vi "slow_control_2_15.vi"() -> ()   [LabVIEW 2018]
uses:
  4623b864-5764-45c6-9cb2-3e18237880ca.vi
  fa57f61f-0bb9-49ac-92eb-fcb40add4dbb.vi
  <vilib>/DAQmx/read.llb/DAQmx Read (Analog 1D DBL NChan 1Samp).vi
  ffb0d1b3-ef19-4e2e-b36e-7277177ef4b3.vi
  9a1acc8a-69db-4048-9e4c-bb07d66d2422.vi
  <vilib>/DAQmx/create/channels.llb/DAQmx Create Channel (AI-Voltage-Basic).vi
  <vilib>/DAQmx/create/channels.llb/DAQmx Create Channel (AI-Current-Basic).vi
  <vilib>/DAQmx/create/channels.llb/DAQmx Create Channel (AI-Temperature-RTD).vi
  <vilib>/DAQmx/miscellaneous.llb/DAQmx Fill In Error Info.vi
  <vilib>/Utility/file.llb/Read Delimited Spreadsheet (string).vi
  <instrlib>/Lake Shore 335/Lake Shore 335.lvlib
  <instrlib>/CAEN PSM/CAEN PSM.lvlib
  <resource>/objmgr/daqmx.rc
panel:
  out "Heater":dbl
  out "Coldhead":dbl
  out "Cycle number":i32
  out "Alarm state":bool
  out "Timestamp last \nmeasured (UPS)":timestamp
  out "Auto-clear":bool
  in  "Auto-clear data?":bool
  in  "Clear data":bool
  in  "Clear data every N cycles":dbl
  in  "N samples":i32=30
  out "Average Flow (SLPM)":dbl caption="Flow (SLPM)"
  out "CAEN Ch. Names":string[](array[string])
  in  "Cycles to execute":dbl=5.0 format="%#_13g"
  out "Detector Pressure":dbl
  in  "N samples":i32=20
  in  "Allows tabs on \nfront panel":T1(tab)
  in  "Anode ch.":enum16{"1", "2", "3", "4"}(ring)=enum."3"
  in  "CAEN unit selector":enum16{"CAEN 1", "CAEN 2"}(ring)
  in  "Multipliers":dbl[](array[numeric])=[1.0, 1.0, 1.0, 1.0, 1.0, 1.0, 1.0, 1.0]
  in  "Offsets\nsubtracted":dbl[](array[numeric])=[0.0, 0.0, 0.0, 0.0, 0.0, 0.0, 0.0, 0.0]
  in  "Channel Names (9207, ai8:15)":string[](array[string])=["i0", "i1", "i2", "i3", "i4", "i5", "i6", "i7"] caption="\"Other\""
  in  "Flow meter input:":u16(ring)=3 items=["v0", "v1", "v2", "v3", "v4", "v5", "v6", "v7"]
  in  "Detector pressure input:":u16(ring) items=["v0", "v1", "v2", "v3", "v4", "v5", "v6", "v7"]
  in  "Channel Names (9207, ai0:7)":string[](array[string])=["v0", "v1", "v2", "v3", "v4", "v5", "v6", "v7"] caption="\"Other\""
  in  "Multipliers":dbl[](array[numeric])=[1.0, 1.0, 1.0, 1.0, 1.0, 1.0, 1.0, 1.0]
  in  "Offsets\nsubtracted":dbl[](array[numeric])=[0.0, 0.0, 0.0, 0.0, 0.0, 0.0, 0.0, 0.0]
  in  "Voltage channels":tag[](array[tag])=["9207/ai0", "9207/ai1", "9207/ai2", "9207/ai3", "9207/ai4", "9207/ai5", "9207/ai6", "9207/ai7"]
  in  "COM-port CAEN 1":refnum<visa-resource-name>
  in  "COM-port CAEN 2":refnum<visa-resource-name>
  in  "Run lakeshore?":bool
  in  "ID Query":bool
  in  "COM-port LakeShore":refnum<visa-resource-name>
  in  "PID settings":cluster{"P":dbl, "I":dbl, "D":dbl}={"P"=50.0, "I"=20.0, "D"=120.0}
  in  "Setpoint (°C)":dbl=-100.0 format="%.1f"
  in  "Heater range":u16(ring) items=["Off", "Low (On)", "Medium", "High"]
  in  "Current channels":tag[](array[tag])=["9207/ai8", "9207/ai9", "9207/ai10", "9207/ai11", "9207/ai12", "9207/ai13", "9207/ai14", "9207/ai15"]
  in  "Channel Names (CAEN)":string[](array[string])=["PMT 1", "PMT 2", "Anode", "Cathode", "Top gate", "Bottom gate", "Other 1", "Other 2"]
  in  "RTD Type":i32(ring)=10071 items=["Pt3750"=12481, "Pt3851"=10071, "Pt3911"=12482, "Pt3916"=10069, "Pt3920"=10053, "Pt3928"=12483, "Custom"=10137]
  in  "Module 1 channels (slot 1)":tag[](array[tag])=["cDAQ2Mod2/ai0", "cDAQ2Mod2/ai1", "cDAQ2Mod2/ai2", "cDAQ2Mod2/ai3", "cDAQ2Mod2/ai4", "cDAQ2Mod2/ai5", "cDAQ2Mod2/ai6", "cDAQ2Mod2/ai7"]
  in  "Current Excitation Source":i32(ring)=10200 items=["Internal"=10200, "External"=10167, "None"=10230]
  in  "Resistance Configuration":i32(ring)=3 items=["2-Wire"=2, "3-Wire"=3, "4-Wire"=4]
  in  "R (T = 0°C):":dbl=100.0
  in  "B":dbl
  in  "A":dbl
  in  "C":dbl
  in  "Module 2 channels (slot 2)":tag[](array[tag])=["cDAQ2Mod3/ai0", "cDAQ2Mod3/ai1", "cDAQ2Mod3/ai2", "cDAQ2Mod3/ai3", "cDAQ2Mod3/ai4", "cDAQ2Mod3/ai5", "cDAQ2Mod3/ai6", "cDAQ2Mod3/ai7"]
  in  "Shut off heater \nif Alarm is active":bool=TRUE
  in  "Re-save headers":bool
  in  "Resistance Configuration":i32(ring)=2 items=["2-Wire"=2, "3-Wire"=3, "4-Wire"=4]
  in  "Module 3 channels":tag[](array[tag])
  in  "RTD Type":i32(ring)=12481 items=["Pt3750"=12481, "Pt3851"=10071, "Pt3911"=12482, "Pt3916"=10069, "Pt3920"=10053, "Pt3928"=12483, "Custom"=10137]
  in  "R (T = 0°C)":dbl=100.0 format="%0.2f"
  out "PT1000 data":dbl[](array[numeric]) format="%0.2f"
  out "9207 (V; A) Converted":dbl[](array[numeric])
  out "9216 #1 (°C)":dbl[](array[numeric])
  out "9216 #2 (°C)":dbl[](array[numeric])
  out "Raw readouts (V, mA)":dbl[](array[numeric]) format="%0.2f"
  out "Det.P input #":i32
  out "Flow input #":i32
  out "PT100 data":dbl[](array[numeric]) format="%0.2f"
  in  "\"Sound\" alarm":bool
  in  "Sound alarm\nFrequency (Hz)":dbl=1680.0
  in  "Send status email now":bool
  out "Email error":i32
  out "source":string
  in  "Number of Bonus lines":i32=1
  out "Names (optional)":string[](array[string])
  in  "Send daily email?":bool=TRUE
  in  "Phone numbers":string[](array[string])
  out "Alarm (or test) message":string
  in  "Alarm\nMaster switch":bool
  in  "Repeat Alarm SMS\nevery N minutes":dbl=15.0
  in  "Test alarm":bool
  out "Warning":bool
  in  "UPS":bool
  in  "UPS Voltage \nLower Threshold":dbl=220.0
  out "NI mod 2&3 status":bool
  in  "NI mod 2&3":bool
  in  "NI mod 1":bool
  in  "CAEN 2":bool
  in  "CAEN 1":bool
  in  "LakeShore":bool
  out "Det. P. warning":bool
  out "Boolean 6":bool
  out "Boolean 5":bool
  out "Boolean 4":bool
  out "Boolean 3":bool
  out "Boolean 2":bool
  out "Boolean":bool
  in  "T 6":bool
  in  "T 5":bool
  in  "T 4":bool
  in  "T 3":bool
  in  "T 2":bool
  in  "T 1":bool
  in  "Detector Pressure":bool
  in  "Overpressure threshold":dbl
  in  "Underpressure threshold":dbl
  out "Comm. status":bool
  in  "High Temp threshold":dbl format="%#_13g"
  in  "Low Temp threshold":dbl format="%#_13g"
  out "LakeShore status":bool
  out "NI mod1 (P) status":bool
  out "CAEN 1 status":bool
  out "CAEN 2 status":bool
  out "Initialization status":bool
  out "Minimum input voltage measured":dbl
  out "Alarm active 2":bool
  out "SMS error":string
  out "Status email preview":string
  in  "Send status email at time:":string="14:00"
  in  "Email Addresses":string[](array[string])
  in  "return address":string="xamsups@gmail.com"
  in  "Ignore Initialization Errors":bool=TRUE caption="Ignore init. errors?"
  out "NI 9226":errorcluster
  in  "HV Channel status":string="Click the button to request the latest High Voltage channel status.\nView another channel with the arrows, or typing 0 through 3."
  out "CAEN 1":T2(array[cluster])
  out "CAEN 2":T2(array[cluster])
  in  "Query HV status":bool
  in  "\"code\"":string="Google this"
  in  "String 7":string="A checkmark means \"No error\" and false. A red X means an error occurred"
  out "\"status\"":bool
  in  "\"source\"":string="This may show two things: the latest executed VI in the task chain, in reverse order, or: which VI produced an error, with a short description. If the error can't easily be resolved, google the code."
  out "NI 9216 x2":errorcluster
  out "CAEN 1":errorcluster
  out "CAEN 2":errorcluster
  out "Lakeshore":errorcluster
  out "NI 9207":errorcluster
  in  "Temperature channel selector":u16(ring) items=["0"=0, "1"=1, "2"=2, "3"=3, "4"=4, "5"=5, "6"=6, "7"=7, "Average"=666]
  out "Heater power (%)":cluster{timestamp[], dbl[]}[](graph)
  out "Flow (SLPM)":cluster{timestamp[], dbl[]}[](graph)
  out "9207 (ai 0:7, Volts)":cluster{timestamp[], dbl[]}[](graph)
  out "Phase Diagram":cluster{"X":dbl, "Y":dbl}[](graph)
  out "Temperature (9216 0:15, °C)":cluster{timestamp[], dbl[]}[](graph)
  in  "Pause?":bool
  out "Integrated Flow (SL)":dbl
  in  "Reset?":bool
  out "LakeShore readings":dbl[](array[numeric])
  out "Detector Temperature (9226, 0:7, °C)":cluster{"X":dbl, "Y":dbl}[](graph)
  out "Temp A":dbl
  out "Temp B":dbl
  in  "Temperature Channel Selector":u16(ring) items=["0", "1", "2", "3", "4", "5", "6", "7"]
  out "Historical Large Phase Diagram":cluster{dbl[], dbl[]}[](graph)
  out "Large Phase Diagram":cluster{"X":dbl, "Y":dbl}[](graph)
  in  "Temperature Channel Selector":u16(ring) items=["0"=0, "1"=1, "2"=2, "3"=3, "4"=4, "5"=5, "6"=6, "7"=7, "Average"=666]
  in  "Scale.Range:Minimum 8":dbl
  in  "Scale.Range:Maximum 8":dbl=4000.0
  in  "Scale.Range:Minimum 7":dbl
  in  "Scale.Range:Maximum 7":dbl=4000.0
  in  "Scale.Range:Minimum 6":dbl=-3000.0
  in  "Scale.Range:Maximum 6":dbl
  in  "Scale.Range:Minimum 5":dbl
  in  "Scale.Range:Maximum 5":dbl=3000.0
  in  "Scale.Range:Minimum 4":dbl=-5000.0
  in  "Scale.Range:Maximum 4":dbl
  in  "Scale.Range:Maximum 3":dbl=4000.0
  in  "Scale.Range:Minimum 3":dbl
  in  "Scale.Range:Maximum 2":dbl=1000.0
  in  "Scale.Range:Minimum 2":dbl
  out "CAEN 1.1":dbl(knob) scale=0.0..1000.0
  out "CAEN 1.1":string
  in  "Scale.Range:Maximum":dbl=1000.0
  in  "Scale.Range:Minimum":dbl
  out "CAEN 2.3 2":string
  out "CAEN 2.2 2":string
  out "Channel Names":string[](array[string])
  out "CAEN 2.3":dbl(knob) scale=0.0..4000.0
  out "CAEN 2.2":dbl(knob) scale=0.0..4000.0
  out "CAEN 2.1":string
  out "CAEN 2.0":string
  out "CAEN 1.3":string
  out "CAEN 1.2":string
  out "CAEN 1.0":string
  out "Channel Names":string[](array[string])
  in  "Set to zero":bool
  out "CAEN 2.1":dbl(knob)
  out "CAEN 2.0":dbl(knob) scale=0.0..3000.0
  in  "Apply Voltage":bool
  in  "VSet (V)":dbl[](array[numeric])
  in  "IMax (uA)":dbl[](array[numeric])
  in  "VMax (V)":dbl[](array[numeric])
  out "CAEN 1.3":dbl(knob)
  out "CAEN 1.2":dbl(knob) scale=0.0..4000.0
  out "CAEN 1.0":dbl(knob) scale=0.0..1000.0
  out "Vmon (V)":dbl[](array[numeric])
  out "IMon (uA)":dbl[](array[numeric])
  in  "Read CAEN units \nevery N cycles":i16=120
  in  "Reset anode\nperiodically?":bool
  in  "Kill every Y minutes":i32=10
  in  "Keep off for X seconds":i32=10
  out "?":bool
  out "Killed":bool
  out "Restarted":bool
  out "Anode timers":timestamp[](array[timestamp])
  out "Seconds until \nanode autokill":dbl format="%.2g"
  out "Seconds until \nanode reset":dbl format="%.2g"
  out "9207 (ai 8:15, Amperes)":cluster{timestamp[], dbl[]}[](graph)
  in  "Kill voltage":bool
  in  "stop":bool
  out "Voltages":dbl[](array[numeric])
  out "Started up?":bool
  out "TOBA appended":dbl[][](array[numeric])
  in  "Read T every N cycles":i32=2
  out "Time until next cycle":dbl format="%.3g"
  in  "Time per cycle (s)":i32=2 caption="Time Target (s)"
  # "<- Proof of concept for New/Old T + New P"
  # "Remove ^this^ array, just for testing and takes up lots of resources"
  # "Moving averages"
  # "NI 9216 Temperature settings"
  # "CAEN settings"
  # "NI 9207 Voltage settings"
  # "If RTD type is custom,\nspecify the Callendar-\nVan Dusen parameters"
  # "Anode connected to:"
  # "Channel:"
  # "NI 9207 Current settings"
  # "Lakeshore settings"
  # "NI 9226 Temperature settings"
  # "Gain (P) (XX.X)"
  # "Reset (I) (XX.X)"
  # "Rate (D) (X.X%)"
  # "Alarm indicators and arms"
  # "Detector Thresholds"
  # "Daily status email"
  # "SMS and sound alarm"
  # "Alarm conditions"
  # "Temperature channels:"
  # "Uninterruptable Power Supply"
  # "Task information"
  # "High Voltage channel status"
  # "How-to"
  # "Data"
  # "Scale:"
  # "to"
  # "to"
  # "Scale:"
  # "Time of last reset"
  # "Time of last reactivation"
  # "to"
  # "Scale:"
  # "to"
  # "Scale:"
  # "Settings"
  # "Scale:"
  # "to"
  # "Scale:"
  # "to"
  # "Scale:"
  # "to"
  # "to"
  # "Scale:"
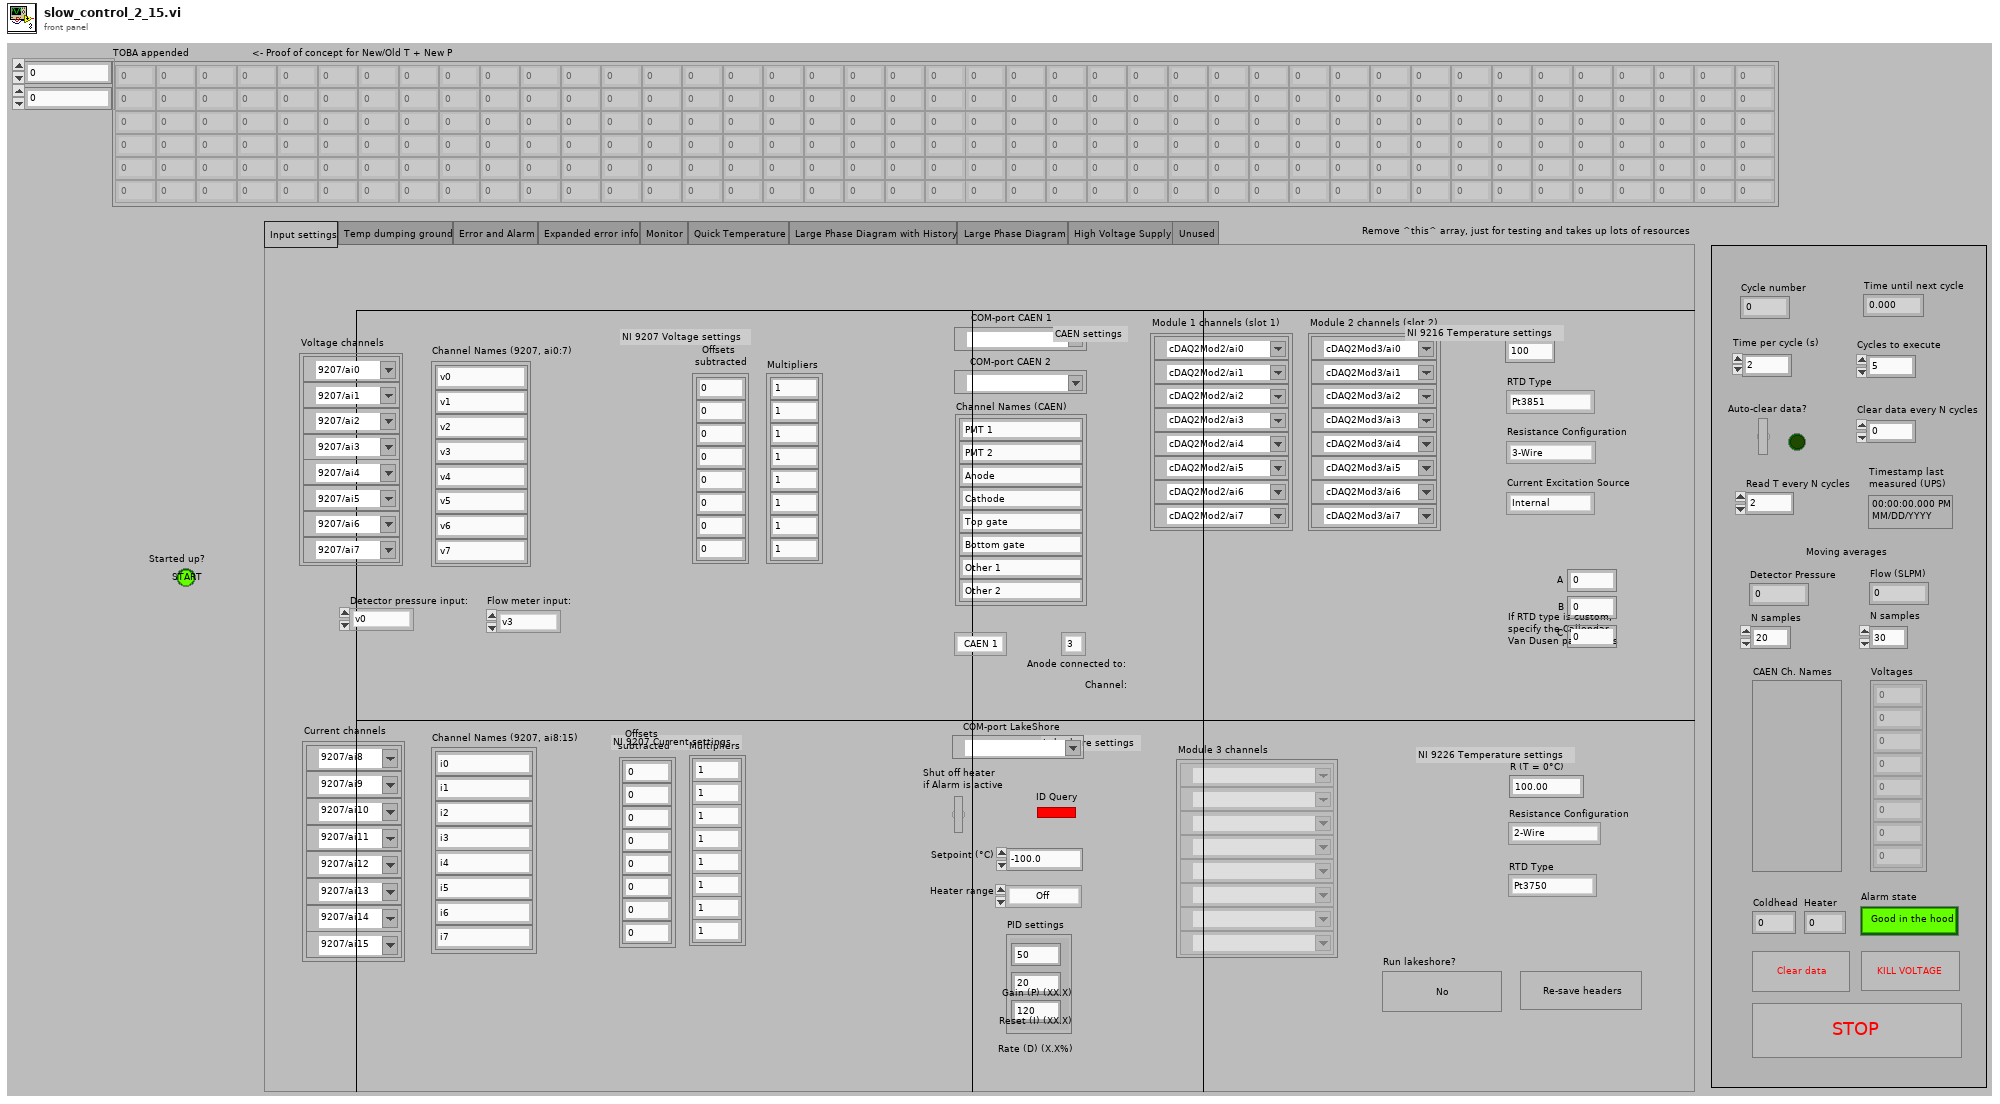
[diagram p1: front panel]
types:
  T1 = enum32{"Input settings", "Temp dumping ground", "Error and Alarm", "Expanded error info", "Monitor", "Quick Temperature", "Large Phase Diagram with History", "Large Phase Diagram", "High Voltage Supply", "Unused"}
  T2 = cluster{"ON":bool, "RUP":bool, "RDW":bool, "OVC":bool, "OVV":bool, "UNV":bool, "MAXV":bool, "TRIP":bool, "OVP":bool, "OVT":bool, "DIS":bool, "KILL":bool, "ILK":bool, "NOCAL":bool}[]
  T3 = cluster{"Baud Rate":u32, "Parity":u16, "Data Bits":u16, "Stop Bits":u16, "Flow Control":u16}
  T4 = cluster{"task out":refnum<k21>, "error out":errorcluster}
  T5 = cluster{"VISA resource name out":refnum<visa-resource-name>, "error out":errorcluster}
  T6 = cluster{"VISA resource name out":refnum<visa-resource-name>, "Board address":u8, "NChannels":u8}
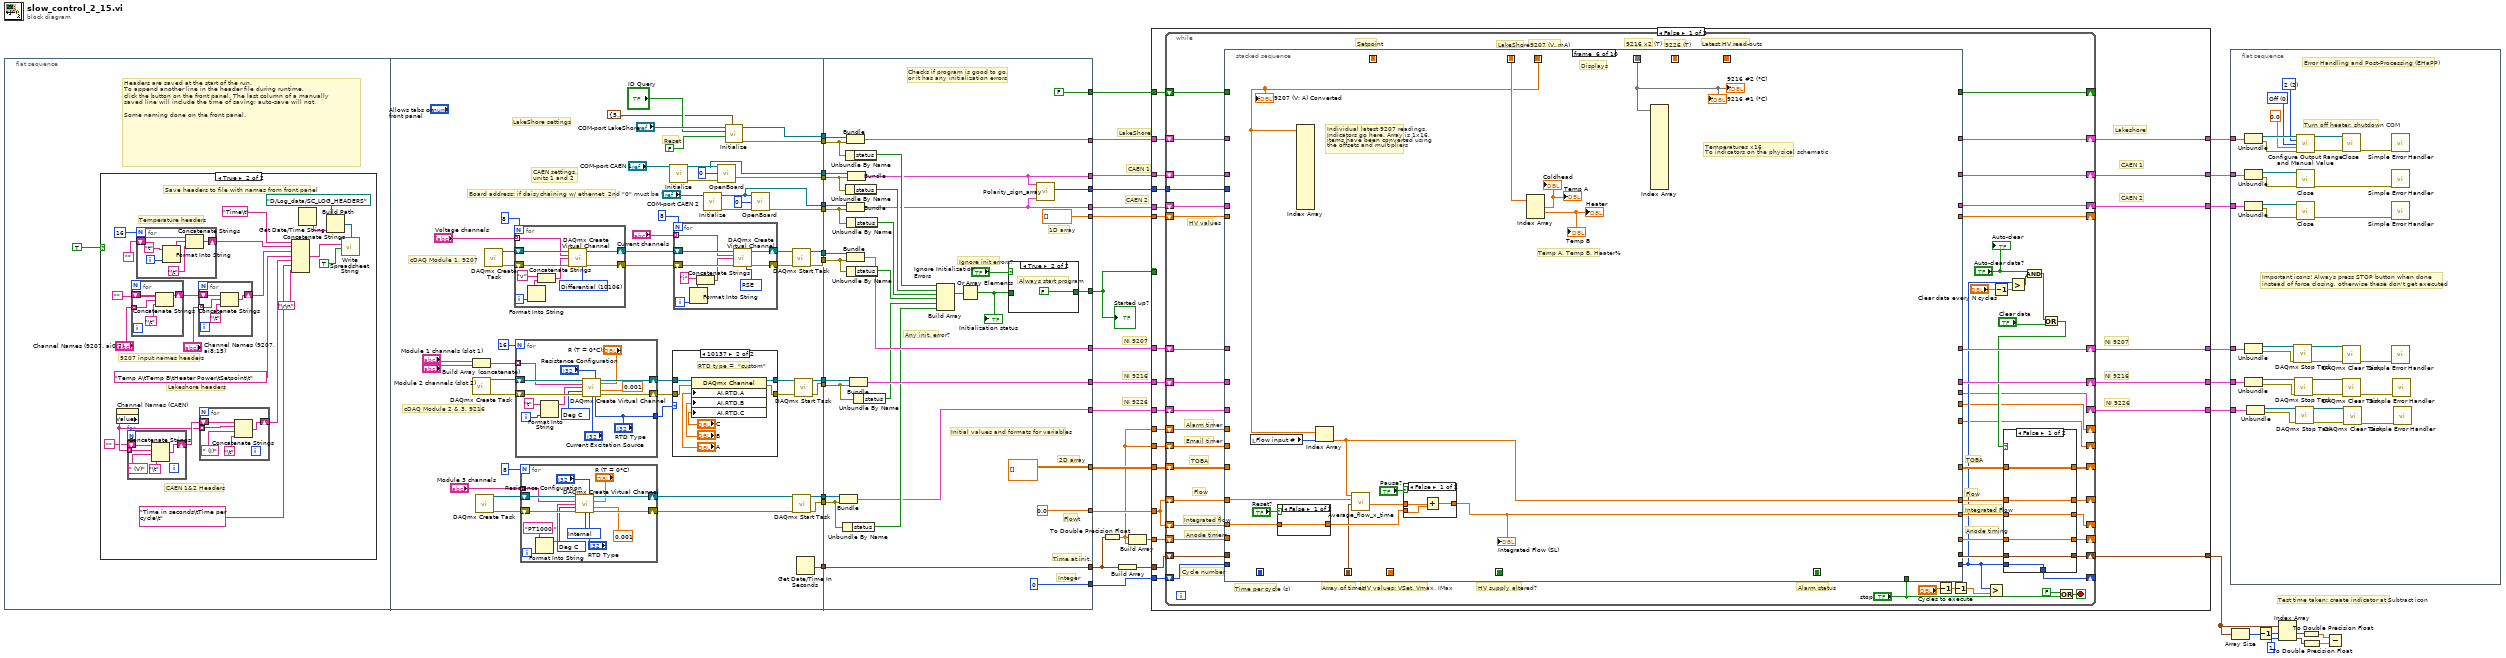
[diagram p0: block diagram]
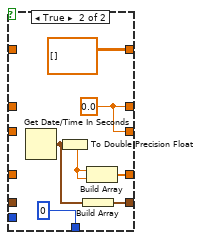
[diagram p2: hidden frame]
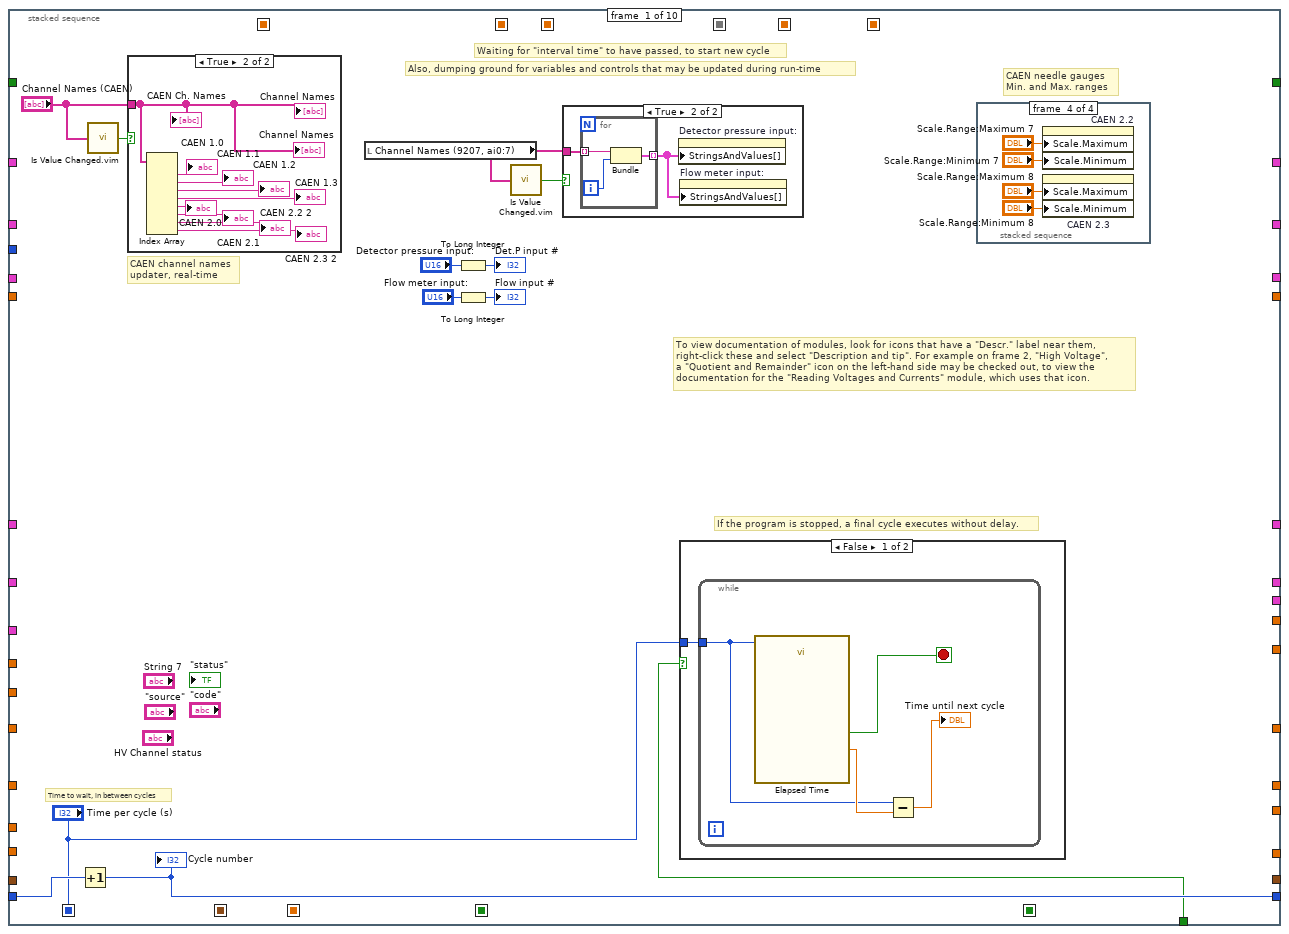
[diagram p3: hidden frame]
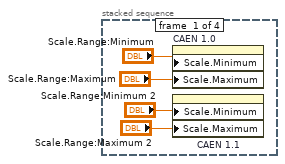
[diagram p6: hidden frame]
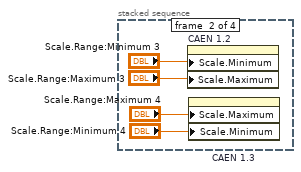
[diagram p7: hidden frame]
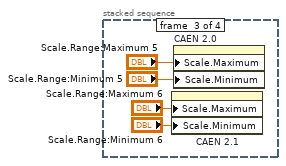
[diagram p8: hidden frame]
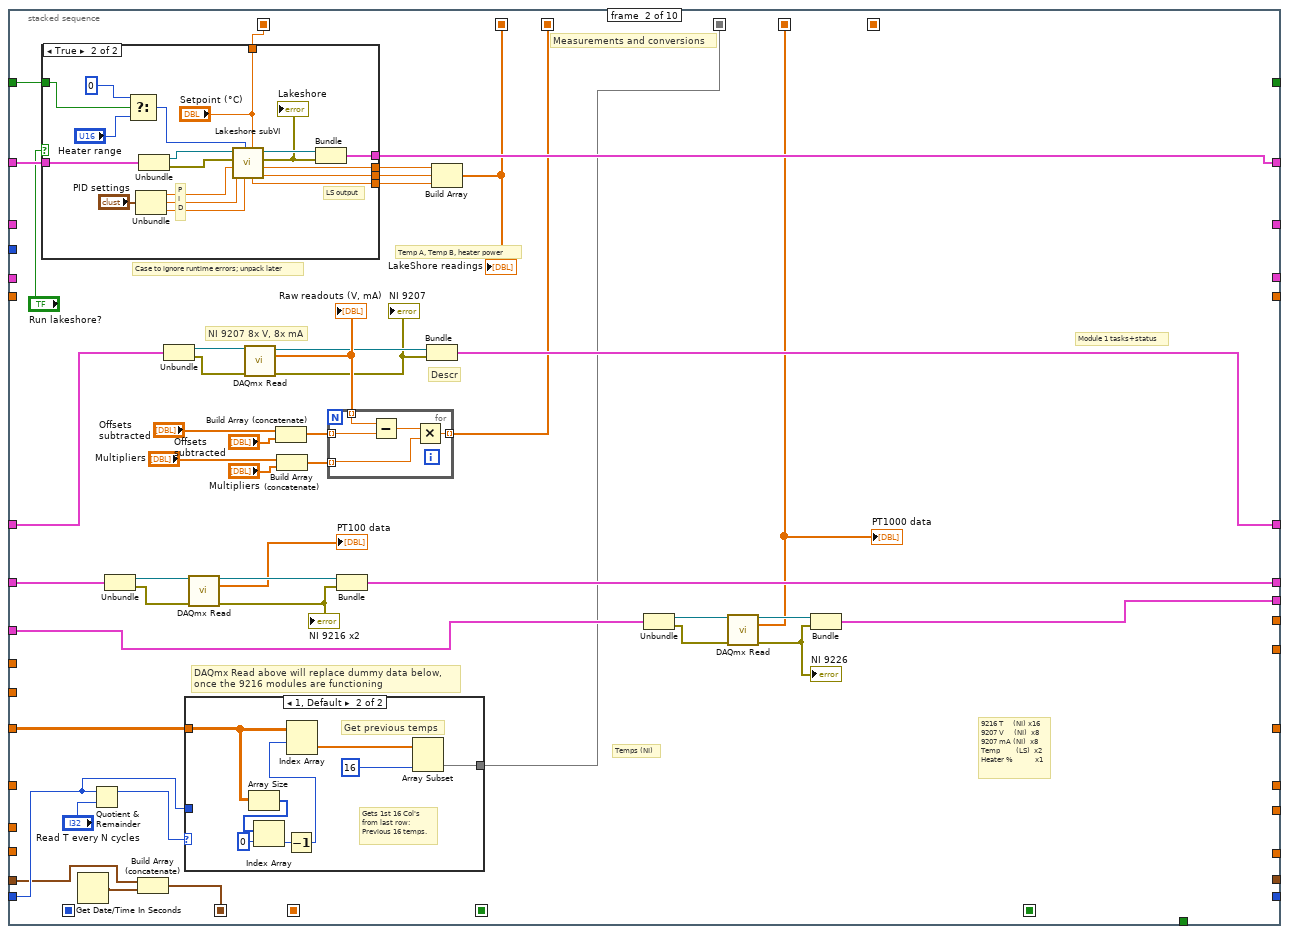
[diagram p10: hidden frame]
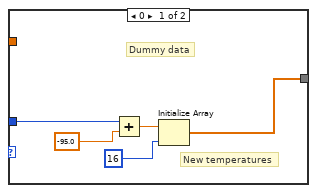
[diagram p11: hidden frame]
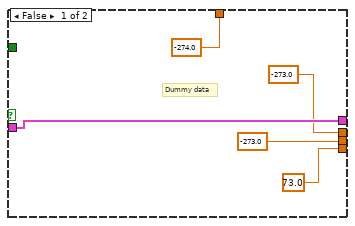
[diagram p12: hidden frame]
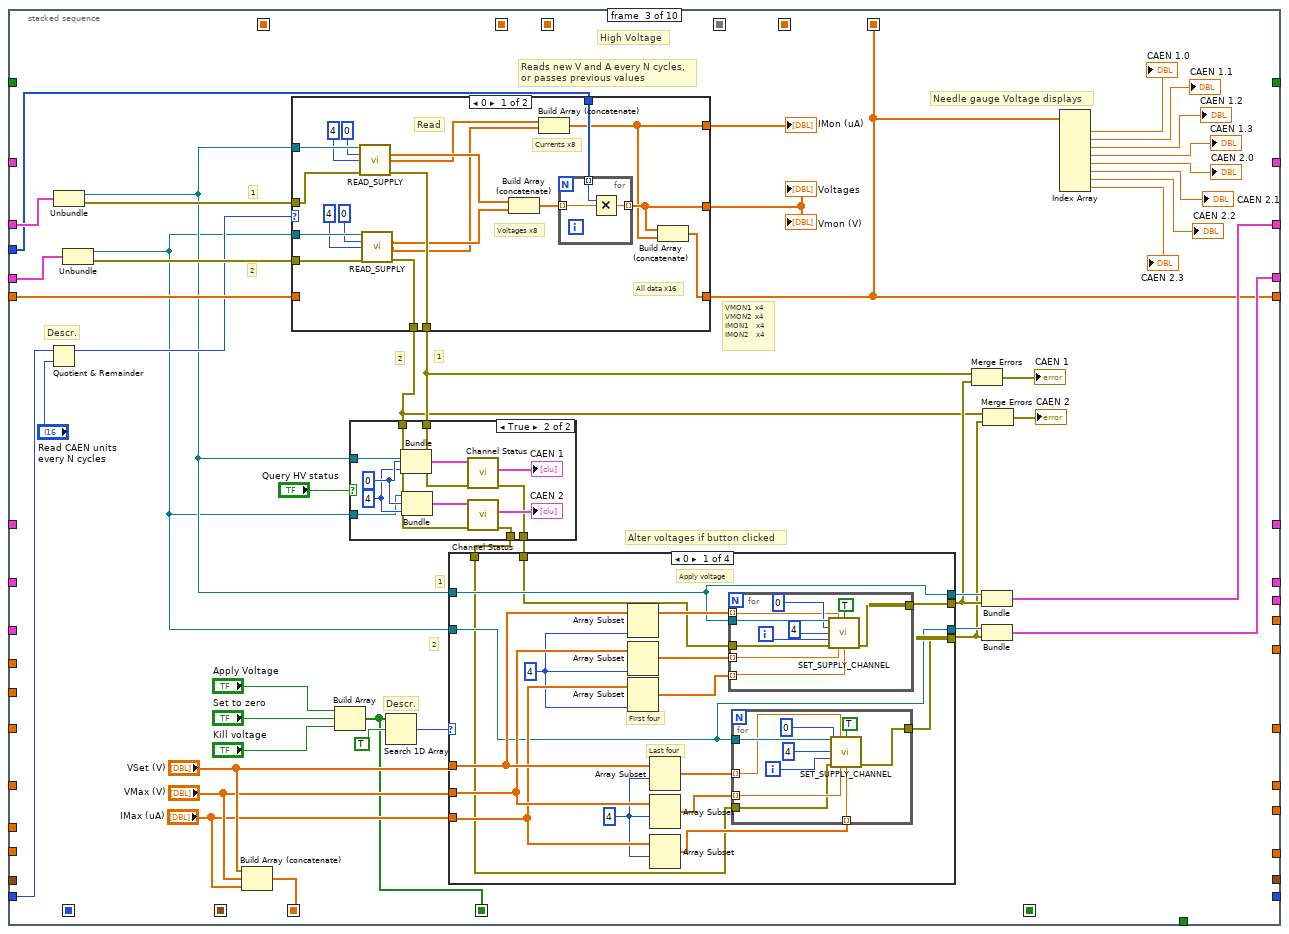
[diagram p13: hidden frame]
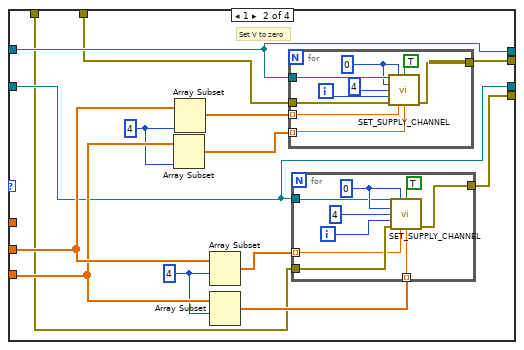
[diagram p15: hidden frame]
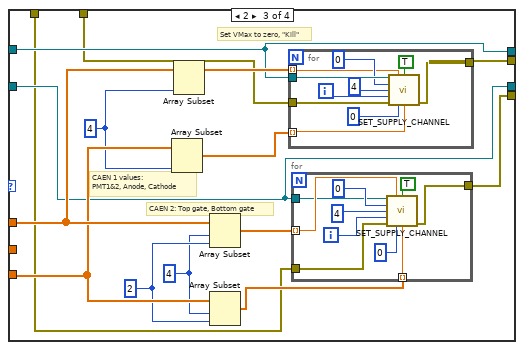
[diagram p16: hidden frame]
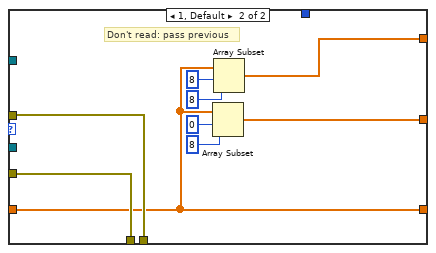
[diagram p18: hidden frame]
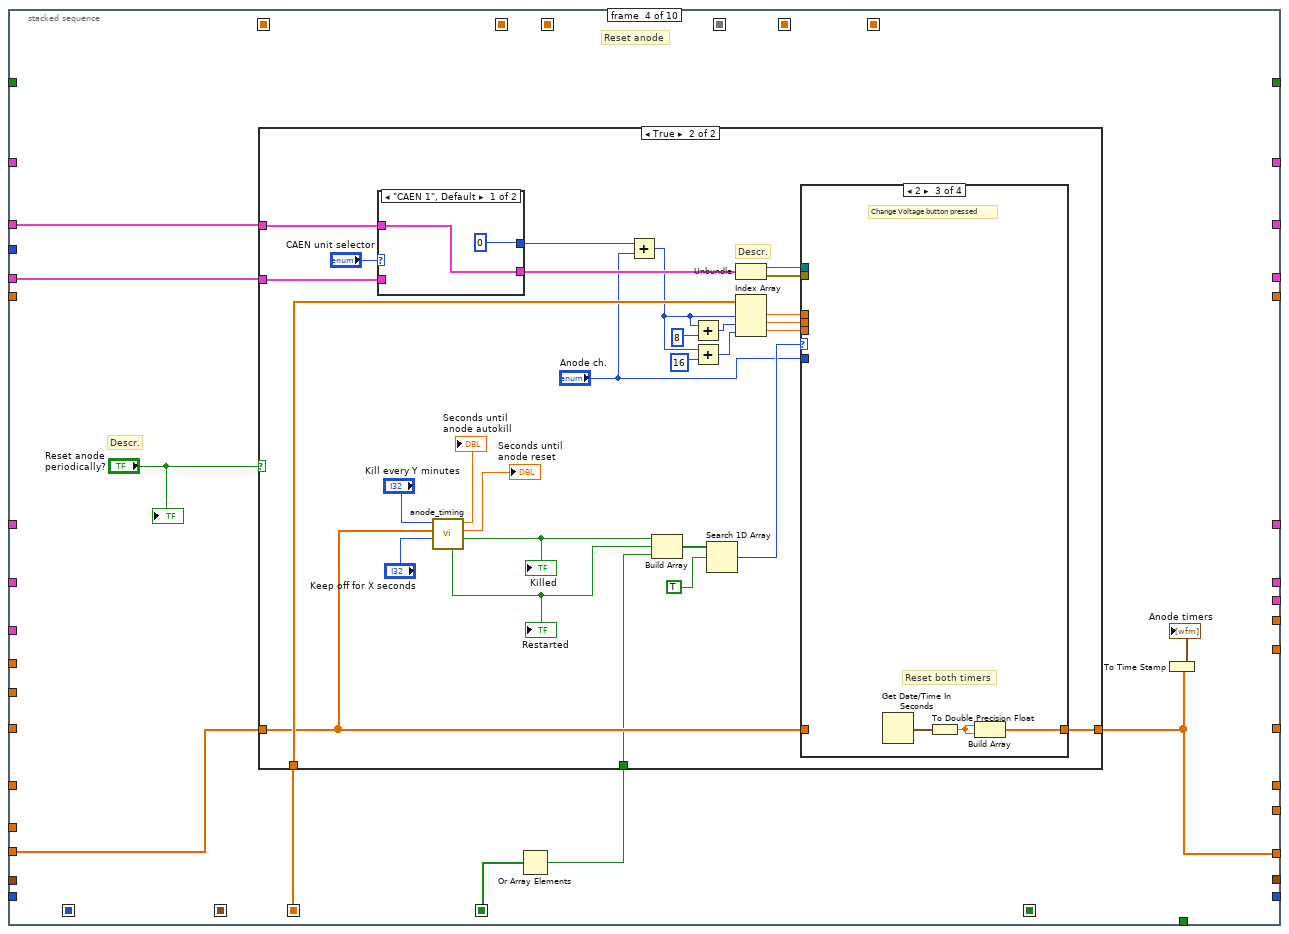
[diagram p19: hidden frame]
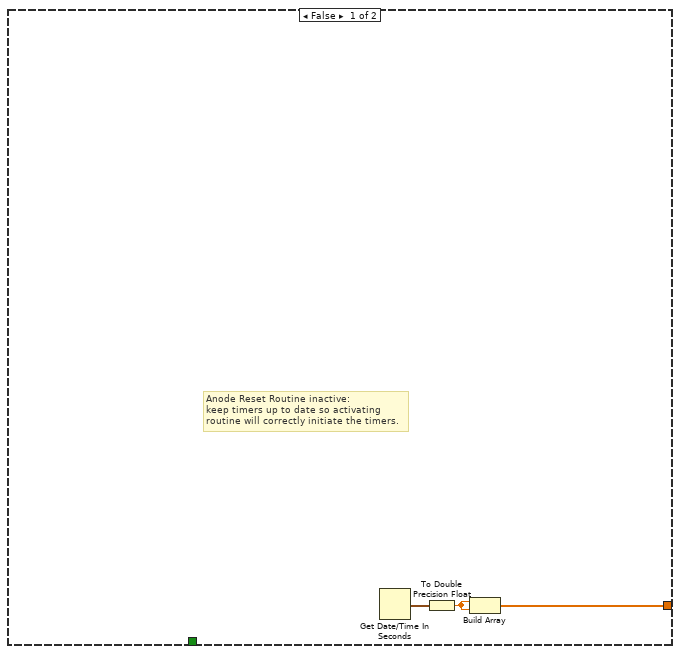
[diagram p20: hidden frame]
diagram:
  # "NI 9226"
  # "NI 9216"
  # "Test time taken: create indicator at Subtract icon"
  # "NI 9207"
  # "CAEN 2"
  # "CAEN 1"
  # "LakeShore"
  n1 = flat-sequence {
    tunnel: [w137] -> w44
    tunnel: [w136] -> w43
    tunnel: [w124] -> w42
    tunnel: [w133] -> w41
    tunnel: [w114] -> w40
    tunnel: [w132] -> w35
    tunnel: [w128] -> w27
    tunnel: [w127] -> w26
    tunnel: [w115] -> w18
    tunnel: [w109] -> w10
    tunnel: [w108] -> w9
    tunnel: [w92] -> w5
    tunnel: [w91] -> w4
    tunnel: w44 -> [w229]
    tunnel: w43 -> [w228]
    tunnel: w42 -> [w226]
    tunnel: w41 -> [w225]
    tunnel: w40 -> [w217]
    tunnel: [w230] -> w24
    tunnel: [0.0] -> w23
    tunnel: [dbl[] []] -> w39
    tunnel: [dbl[][] []] -> w11
    tunnel: [0] -> w38
    tunnel: [w227] -> w37
    tunnel: [w200] -> w36
    tunnel: [w224] -> w22
    tunnel: w35 -> [w224]
    tunnel: w27 -> [w222]
    tunnel: w26 -> [w221]
    tunnel: [w199] -> w25
    tunnel: [FALSE] -> w19
    tunnel: w18 -> [w218]
    tunnel: [w216] -> w17
    tunnel: w10 -> [w209]
    tunnel: w9 -> [w208]
    tunnel: [w207] -> w8
    tunnel: w5 -> [w204]
    tunnel: w4 -> [w203]
    tunnel: [w201] -> w3
    tunnel: [w198] -> w1
    frame #0 {
      # "Headers are saved at the start of the run.\nTo append another line in the header file during runtime,\nclick the button on the front panel. The last column of a manually\nsaved line will include the time of saving; auto-save will not.\n\nSome naming done on the front panel."
      n2 = case shown="True" TRUE {
        frame False {
        }
        frame True {
          # "CAEN 1&2 Headers"
          # "Lakeshore headers"
          # "9207 input names headers"
          # "Temperature headers"
          # "Save headers to file with names from front panel"
          n3 = property on="Channel Names (CAEN)" class="Arr (strict)"() -> ("Value"=w51:string[])  [unwired: 2 in, 2 out]
          n4 = for {
            tunnel: w51 -> [w75] mode=indexing
            shift-right: [w73] -> w52
            shift-left: "" -> [w72]
            n5 = Concatenate Strings(w72, w75, " (V)", "\t") -> (w73:string)
          }
          n6 = for {
            shift-right: [w83] -> w55
            shift-left: "" -> [w84]
            tunnel: "Channel Names (9207, ai0:7)" -> [w81] mode=indexing
            n7 = Concatenate Strings(w84, w81, "\t") -> (w83:string)
          }
          n8 = for {
            N: 16 -> [_]
            shift-right: [w85] -> w58
            shift-left: "" -> [w86]
            i -> [w90]
            n9 = Format Into String(initial string="t", w90) -> (resulting string=w88:string)  [unwired: 2 in, 1 out]
            n10 = Concatenate Strings(w86, w88, "\t") -> (w85:string)
          }
          n11 = for {
            shift-right: [w78] -> w54
            shift-left: w55 -> [w80]
            tunnel: "Channel Names (9207, ai8:15)" -> [w77] mode=indexing
            n12 = Concatenate Strings(w80, w77, "\t") -> (w78:string)
          }
          n13 = for {
            shift-right: [w68] -> w50
            shift-left: w52 -> [w69]
            tunnel: w51 -> [w67] mode=indexing
            n14 = Concatenate Strings(w69, w67, " (I)", "\t") -> (w68:string)
          }
          n15 = Concatenate Strings("Time\t", w58, w54, "Temp A\tTemp B\tHeater Power\tSetpoint\t", w50, "Time in seconds\tTime per cycle\t", "\r\n") -> (w57:string)
          n16 = Get Date/Time String() -> (date string=w61:string)  [unwired: 3 in, 1 out]
          n17 = Build Path(base path=path "D:/Log_data/SC_LOG_HEADERS" ("file path (dialog if empty)"), name or relative path=w61) -> (appended path=w62:path)
          n18 = call <vilib>:"Write Spreadsheet String.vi"("append to file? (new file:F)"=TRUE, "spreadsheet string"=w57, "file path (dialog if empty)"=w62) -> ()  [unwired: 7 in, 2 out]
        }
      }
    }
    frame #1 {
      # "cDAQ Module 2 & 3, 9216"
      # "cDAQ Module 1, 9207"
      # "Board address: if daisychaining w/ ethernet, 2nd \"0\" must be \"1\""
      # "CAEN settings,\nunits 1 and 2"
      # "Reset"
      # "LakeShore settings"
      n19 = call <vilib>:"DAQmx Create Task.vi"() -> ("task out"=w107:refnum<k21>, "error out"=w110:errorcluster)  [unwired: 14 in]
      n20 = Build Array (concatenate)("Module 1 channels (slot 1)", "Module 2 channels (slot 2)") -> (w104:tag[])
      n21 = call <vilib>:"DAQmx Create Task.vi"() -> ("task out"=w97:refnum<k21>, "error out"=w96:errorcluster)  [unwired: 14 in]
      n22 = call <vilib>:"DAQmx Create Task.vi"() -> ("task out"=w123:refnum<k21>, "error out"=w122:errorcluster)  [unwired: 14 in]
      n23 = for {
        N: 8 -> [_]
        shift-right: [w193] -> w119
        shift-left: w123 -> [w192]
        shift-right: [w194] -> w118
        shift-left: w122 -> [w190]
        tunnel: "Voltage channels" -> [w191] mode=indexing
        i -> [w196]
        w188 = 10106 items=["Default"=-1, "RSE"=10083, "NRSE"=10078, "Differential"=10106, "Pseudodifferential"=12529] ("input terminal configuration")
        n24 = Format Into String(w196) -> (resulting string=w195:string)  [unwired: 3 in, 1 out]
        n25 = Concatenate Strings("v" ("string"), w195) -> (w189:string)
        n26 = call-poly <vilib>:"DAQmx Create Virtual Channel.vi"("task in"=w192, "input terminal configuration"=w188, "physical channels"=w191, "name to assign"=w189, "error in"=w190) -> ("task out"=w193:refnum<k21>, "error out"=w194:errorcluster)  [unwired: 9 in]
      }
      n27 = for {
        N: 16 -> [_]
        shift-right: [w174] -> w103
        shift-left: w107 -> [w177]
        shift-right: [w175] -> w102
        shift-left: w110 -> [w176]
        tunnel: w104 -> [w173] mode=indexing
        tunnel: ["RTD Type"] -> w99
        i -> [w171]
        w168 = 10143 items=["Deg C"=10143, "Deg F"=10144, "Kelvins"=10325, "Deg R"=10145, "From Custom Scale"=10065] ("units")
        n28 = Format Into String(initial string="t", w171) -> (resulting string=w170:string)  [unwired: 2 in, 1 out]
        n29 = call-poly <vilib>:"DAQmx Create Virtual Channel.vi"("task in"=w177, "resistance configuration"="Resistance Configuration", "physical channels"=w173, "r0"="R (T = 0°C):", "name to assign"=w170, "units"=w168, "current excitation value"=0.001, "error in"=w176, "current excitation source"="Current Excitation Source", "rtd type"="RTD Type") -> ("task out"=w174:refnum<k21>, "error out"=w175:errorcluster)  [unwired: 4 in]
      }
      n30 = for {
        N: 8 -> [_]
        shift-right: [w152] -> w94
        shift-left: w97 -> [w151]
        shift-right: [w153] -> w93
        shift-left: w96 -> [w154]
        tunnel: "Module 3 channels" -> [w149] mode=indexing
        i -> [w147]
        w143 = 10200 items=["Internal"=10200, "External"=10167, "None"=10230] ("current excitation source")
        w145 = 10143 items=["Deg C"=10143, "Deg F"=10144, "Kelvins"=10325, "Deg R"=10145, "From Custom Scale"=10065] ("units")
        n31 = Format Into String(initial string="PT1000.", w147) -> (resulting string=w146:string)  [unwired: 2 in, 1 out]
        n32 = call-poly <vilib>:"DAQmx Create Virtual Channel.vi"("task in"=w151, "resistance configuration"="Resistance Configuration", "physical channels"=w149, "r0"="R (T = 0°C)", "name to assign"=w146, "units"=w145, "current excitation value"=0.001, "error in"=w154, "current excitation source"=w143, "rtd type"="RTD Type") -> ("task out"=w152:refnum<k21>, "error out"=w153:errorcluster)  [unwired: 4 in]
      }
      n33 = call <instrlib>:"Initialize.vi"("VISA resource name"="COM-port CAEN 1") -> ("error out"=w134:errorcluster, "VISA resource name out"=w124:refnum<visa-resource-name>)  [unwired: 9 in]
      n34 = case shown="10137" w99 {
        tunnel: w103 -> [w156 w160]
        tunnel: w102 -> [w155 w159]
        tunnel: [w156 w158] -> w101
        tunnel: [w155 w157] -> w100
        frame 0, Default {
          # "Don't need to specify the A, B, C\nvalues if RTD type is not \"custom\""
        }
        frame 10137 {
          # "RTD type =  \"custom\""
          n35 = property class="DAQmx Channel"(reference=w160, error in=w159, "AI.RTD.A"="A", "AI.RTD.B"="B", "AI.RTD.C"="C") -> (reference out=w158:refnum<k21>, error out=w157:errorcluster)
        }
      }
      n36 = for {
        N: 8 -> [_]
        shift-right: [w179] -> w116
        shift-left: w119 -> [w186]
        shift-right: [w178] -> w117
        shift-left: w118 -> [w185]
        tunnel: "Current channels" -> [w184] mode=indexing
        i -> [w183]
        w187 = 10083 items=["default"=-1, "RSE"=10083, "NRSE"=10078, "Differential"=10106, "Pseudodifferential"=12529] ("input terminal configuration")
        n37 = Format Into String(w183) -> (resulting string=w181:string)  [unwired: 3 in, 1 out]
        n38 = Concatenate Strings("i", w181) -> (w180:string)
        n39 = call-poly <vilib>:"DAQmx Create Virtual Channel.vi"("task in"=w186, "input terminal configuration"=w187, "physical channels"=w184, "name to assign"=w180, "error in"=w185) -> ("task out"=w179:refnum<k21>, "error out"=w178:errorcluster)  [unwired: 9 in]
      }
      n40 = call <instrlib>:"Initialize.vi"("VISA resource name"="COM-port CAEN 2") -> ("error out"=w129:errorcluster, "VISA resource name out"=w128:refnum<visa-resource-name>)  [unwired: 9 in]
      n41 = call <instrlib>:"OpenBoard.vi"("error in (no error)"=w134, "Board Address"=0, "VISA resource name"=w124) -> ("error out"=w133:errorcluster)  [unwired: 7 in, 1 out]
      n42 = call <instrlib>:"Initialize.vi"("Serial Configuration"=T3 {"Baud Rate"=57600, "Parity"=1, "Data Bits"=7, "Stop Bits"=10, "Flow Control"=0}, "Reset (True)"=FALSE ("Reset (LakeShore)"), "ID Query (True)"="ID Query", "VISA resource name"="COM-port LakeShore") -> ("error out"=w136:errorcluster, "VISA resource name out"=w137:refnum<visa-resource-name>)  [unwired: 6 in]
      n43 = call <instrlib>:"OpenBoard.vi"("error in (no error)"=w129, "Board Address"=u8 0, "VISA resource name"=w128) -> ("error out"=w127:errorcluster)  [unwired: 7 in, 1 out]
      n44 = call <vilib>:"DAQmx Start Task.vi"("task/channels in"=w116, "error in"=w117) -> ("task out"=w115:refnum<k21>, "error out"=w114:errorcluster)  [unwired: 12 in]
      n45 = call <vilib>:"DAQmx Start Task.vi"("task/channels in"=w94, "error in"=w93) -> ("task out"=w92:refnum<k21>, "error out"=w91:errorcluster)  [unwired: 12 in]
      n46 = call <vilib>:"DAQmx Start Task.vi"("task/channels in"=w101, "error in"=w100) -> ("task out"=w109:refnum<k21>, "error out"=w108:errorcluster)  [unwired: 12 in]
      n47 = Get Date/Time In Seconds() -> (seconds since 1Jan1904=w132:timestamp)
    }
    frame #2 {
      # "1D array"
      # "Initial values and formats for variables"
      # "Time at init."
      # "Integer"
      # "2D array"
      # "Flowt"
      # "Checks if program is good to go,\nor it has any initialization errors"
      # "Ignore init errors?"
      # "Any init. error?"
      n48 = Bundle("task out"=w204, "error out"=w203) -> (w201:T4)  [unwired: 1 in]
      n49 = Unbundle By Name(w203) -> ("status"=w202:bool)
      n50 = Unbundle By Name(w225) -> ("status"=w231:bool)
      n51 = Unbundle By Name(w228) -> ("status"=w210:bool)
      n52 = Bundle("VISA resource name out"=w229, "error out"=w228) -> (w227:T5)  [unwired: 1 in]
      n53 = Unbundle By Name(w221) -> ("status"=w223:bool)
      n54 = Unbundle By Name(w217) -> ("status"=w211:bool)
      n55 = Bundle("VISA resource name out"=w222, "error out"=w221) -> (w199:T5)  [unwired: 1 in]
      n56 = Bundle("task out"=w218, "error out"=w217) -> (w216:T4)  [unwired: 1 in]
      n57 = Bundle("VISA resource name out"=w226, "error out"=w225) -> (w200:T5)  [unwired: 1 in]
      n58 = Bundle("task out"=w209, "error out"=w208) -> (w207:T4)  [unwired: 1 in]
      n59 = Unbundle By Name(w208) -> ("status"=w206:bool)
      n60 = Build Array(w210, w231, w211, w223, w206, w202) -> (w232:bool[])
      n61 = Or Array Elements(Boolean array=w232) -> (logical OR=w205:bool)
      "Initialization status" <- w205
      n62 = case shown="True" "Ignore Initialization Errors" {
        tunnel: [w233 FALSE] -> w230
        tunnel: w205 -> [w233 _]
        frame False {
          # "Only start if no errors"
        }
        frame True {
          # "Always start program"
        }
      }
      n63 = call "Polarity_sign_array.vi"("CAEN 2 in"=w199, "CAEN 1 in"=w200) -> ("Polarity signs"=w198:i32[])  [unwired: 7 in, 2 out]
    }
  }
  n64 = To Double Precision Float(number=w22) -> (double precision float=w6:dbl)
  n65 = Build Array(w22) -> (w34:timestamp[])
  n66 = Build Array(w6, w6) -> (w21:dbl[])
  n67 = case shown="False" w24 {
    selector: w24 -> [_ w1160]
    tunnel: [_ w1160] -> _
    tunnel: w39 -> [w250 _]
    tunnel: w38 -> [w257 _]
    tunnel: w11 -> [w256 _]
    tunnel: w37 -> [w251 w1158]
    tunnel: w36 -> [w253 w1157]
    tunnel: w34 -> [w255 _]
    tunnel: [w254 timestamp[] []] -> w30
    tunnel: w25 -> [w252 w1156]
    tunnel: w23 -> [w246 _]
    tunnel: w21 -> [w249 _]
    tunnel: [w248 w1158] -> w20
    tunnel: w19 -> [w247 _]
    tunnel: w17 -> [w245 w1155]
    tunnel: [w244 w1157] -> w16
    tunnel: [w243 w1156] -> w15
    tunnel: [w242 w1155] -> w14
    tunnel: w8 -> [w241 w1154]
    tunnel: [w240 w1154] -> w7
    tunnel: w6 -> [w239 _]
    tunnel: w6 -> [w238 _]
    tunnel: w3 -> [w237 w1153]
    tunnel: [w236 w1153] -> w2
    tunnel: w1 -> [w235 _]
    frame False {
      # "NI 9226"
      # "NI 9216"
      # "NI 9207"
      # "CAEN 2"
      # "CAEN 1"
      # "Lakeshore"
      n68 = while {
        shift-right: [w271] -> _
        shift-left: w257 -> [w309]
        shift-right: [w284] -> _
        shift-left: w256 -> [w298]
        shift-right: [w276] -> w254
        shift-left: w255 -> [w306]
        shift-right: [w300] -> w244
        shift-left: w253 -> [w293]
        shift-right: [w302] -> _
        shift-left: w250 -> [w305]
        shift-right: [w299] -> w243
        shift-left: w252 -> [w304]
        shift-right: [w301] -> w248
        shift-left: w251 -> [w303]
        shift-right: [w280] -> _
        shift-left: w246 -> [w295]
        shift-right: [w282] -> _
        shift-left: w246 -> [w296]
        shift-right: [w278] -> _
        shift-left: w249 -> [w294]
        shift-right: [w266] -> _
        shift-left: w247 -> [w292]
        shift-right: [w290] -> w242
        shift-left: w245 -> [w291]
        shift-right: [w288] -> w240
        shift-left: w241 -> [w289]
        shift-right: [w264] -> _
        shift-left: w239 -> [w265]
        shift-right: [w261] -> _
        shift-left: w238 -> [w262]
        shift-right: [w259] -> w236
        shift-left: w237 -> [w260]
        tunnel: w235 -> [w258]
        stop <- w307 stop-if-true
        # "9226 (T)"
        # "Email timer"
        # "Alarm timer"
        # "Alarm status"
        # "LakeShore"
        # "9216 x2 (T)"
        # "9207 (V, mA)"
        # "HV supply altered?"
        # "Setpoint"
        # "Anode timing"
        # "Anode timers"
        # "Integrated flow"
        # "Flow"
        # "Flow"
        # "Integrated Flow"
        # "TOBA"
        # "Array of times"
        # "Latest HV read-outs"
        # "Time per cycle (s)"
        # "Cycle number"
        # "HV values: VSet, Vmax, IMax"
        # "HV values"
        # "TOBA"
        n69 = stacked-sequence {
          seq-local: [_ _ w477 _ _ _ _ _ _ _] -> [_ _ _ w660 _ _ _ _ _ _]
          seq-local: ["Time per cycle (s)" _ _ _ _ _ _ _ _ _] -> [_ _ _ _ _ _ w861 _ _ _]
          seq-local: [_ _ w468 _ _ _ _ _ _ _] -> [_ _ _ _ _ _ w863 _ _ _]
          seq-local: [_ w410 _ _ _ _ _ _ _ _] -> [_ _ _ _ w735 w844 _ _ _ _]
          seq-local: [_ _ w471 _ _ _ _ _ _ _] -> [_ _ _ w655 _ _ _ _ _ _]
          seq-local: [_ w403 _ _ _ _ _ _ _ _] -> [_ _ _ _ _ _ w877 _ _ _]
          seq-local: [_ w398 _ _ _ _ _ _ _ _] -> [_ _ _ _ w747 w836 w865 w965 w997 w1082]
          seq-local: [_ w370 _ _ _ _ _ _ _ _] -> [_ _ _ _ w750 w839 w857 _ _ _]
          seq-local: [_ w386 _ _ _ _ _ _ _ _] -> [_ _ _ _ w749 w838 w864 _ _ _]
          seq-local: [_ _ _ _ _ _ _ w925 _ _] -> [_ _ _ _ _ _ _ _ w999 w1083]
          seq-local: [_ w371 _ _ _ _ _ _ _ _] -> [_ _ _ _ w733 _ w856 w923 w993 w1065]
          tunnel: [w333 _ _ _ _ _ _ _ _ _] -> w270
          tunnel: "stop" -> [w332 _ _ _ _ _ _ _ _ _]
          tunnel: w309 -> [w334 w399 w493 _ _ _ _ _ _ _]
          tunnel: w298 -> [_ w400 _ _ w779 _ _ _ _ _]
          tunnel: [_ _ _ _ w736 _ _ _ _ _] -> w285
          tunnel: w306 -> [_ w378 _ _ _ _ _ _ _ _]
          tunnel: w293 -> [_ _ w500 w661 _ _ _ w981 _ _]
          tunnel: w305 -> [_ _ w498 _ _ _ _ _ _ _]
          tunnel: w304 -> [_ _ w497 w656 _ _ _ w980 _ _]
          tunnel: w303 -> [_ w412 _ _ _ _ _ w979 _ _]
          tunnel: [_ w413 _ _ _ _ _ _ _ _] -> w301
          tunnel: [_ _ w468 _ _ _ _ _ _ _] -> w302
          tunnel: [_ _ w483 _ _ _ _ _ _ _] -> w300
          tunnel: [_ _ w481 _ _ _ _ _ _ _] -> w299
          tunnel: [_ _ _ _ w735 _ _ _ _ _] -> w277
          tunnel: w295 -> [_ _ _ _ _ w842 _ _ _ _]
          tunnel: w296 -> [_ _ _ _ _ w843 _ _ _ _]
          tunnel: w294 -> [_ _ _ w662 _ _ _ _ _ _]
          tunnel: [_ _ _ w657 _ _ _ _ _ _] -> w279
          tunnel: w292 -> [_ w406 _ _ _ _ _ _ _ _]
          tunnel: w291 -> [_ w405 _ _ _ _ _ w978 _ _]
          tunnel: [_ w401 _ _ _ _ _ _ _ _] -> w290
          tunnel: [_ _ _ _ _ w841 _ _ _ _] -> w281
          tunnel: [_ _ _ _ _ w840 _ _ _ _] -> w283
          tunnel: w289 -> [_ w385 _ _ _ _ _ w966 _ _]
          tunnel: [_ w380 _ _ _ _ _ _ _ _] -> w288
          tunnel: [_ _ _ _ _ _ _ _ w1001 _] -> w266
          tunnel: w265 -> [_ _ _ _ _ _ _ _ w996 _]
          tunnel: [_ _ _ _ _ _ _ _ w994 _] -> w264
          tunnel: w262 -> [_ _ _ _ _ _ _ _ _ w1070]
          tunnel: [_ _ _ _ _ _ _ _ _ w1069] -> w261
          tunnel: w260 -> [_ w377 _ _ _ _ _ _ _ _]
          tunnel: [_ w372 _ _ _ _ _ _ _ _] -> w259
          tunnel: w258 -> [_ _ w462 _ _ _ _ _ _ _]
          frame #0 {
            # "CAEN channel names\nupdater, real-time"
            # "Also, dumping ground for variables and controls that may be updated during run-time"
            # "CAEN needle gauges\nMin. and Max. ranges"
            # "To view documentation of modules, look for icons that have a \"Descr.\" label near them,\nright-click these and select \"Description and tip\". For example on frame 2, \"High Voltage\",\na \"Quotient and Remainder\" icon on the left-hand side may be checked out, to view the\ndocumentation for the \"Reading Voltages and Currents\" module, which uses that icon."
            # "Time to wait, in between cycles"
            # "If the program is stopped, a final cycle executes without delay."
            # "Waiting for \"interval time\" to have passed, to start new cycle"
            n70 = Increment(x=w334) -> (x+1=w333:i32)
            "Cycle number" <- w333
            n71 = call "Is Value Changed.vim"("value"="Channel Names (CAEN)") -> ("changed or first call?"=w325:bool)
            n72 = case shown="True" w325 {
              tunnel: "Channel Names (CAEN)" -> [_ w340]
              frame False {
              }
              frame True {
                n73 = Index Array(array=w340) -> (element #1=→"CAEN 1.0":string, element #2=→"CAEN 1.1":string, element #3=→"CAEN 1.2":string, element #4=→"CAEN 1.3":string, element #5=→"CAEN 2.0":string, element #6=→"CAEN 2.1":string, element #7=→"CAEN 2.2 2":string, element #8=→"CAEN 2.3 2":string)  [unwired: 8 in]
                "CAEN Ch. Names" <- w340
                "Channel Names" <- w340
                "Channel Names" <- w340
              }
            }
            n74 = local read "Channel Names (9207, ai0:7)"() -> (w323:string[])
            n75 = To Long Integer(number="Detector pressure input:") -> (32bit integer=→"Det.P input #":i32)
            n76 = To Long Integer(number="Flow meter input:") -> (32bit integer=→"Flow input #":i32)
            n77 = call "Is Value Changed.vim"("value"=w323) -> ("changed or first call?"=w324:bool)
            n78 = case shown="True" w324 {
              tunnel: w323 -> [_ w336]
              frame False {
                # ":D"
              }
              frame True {
                n79 = for {
                  tunnel: w336 -> [w339] mode=indexing
                  tunnel: [w337] -> w335 mode=indexing
                  i -> [w338]
                  n80 = Bundle("Or give name if \"Other\""=w339, w338) -> (w337:cluster{"Or give name if \"Other\"":string, i32})  [unwired: 1 in]
                }
                n81 = property on="Detector pressure input:" class="Ring (strict)"("StringsAndValues[]"=w335) -> ()  [unwired: 2 in, 2 out]
                n82 = property on="Flow meter input:" class="Ring (strict)"("StringsAndValues[]"=w335) -> ()  [unwired: 2 in, 2 out]
              }
            }
            n83 = case shown="False" w332 {
              tunnel: "Time per cycle (s)" -> [w365 _]
              frame False {
                n84 = while {
                  tunnel: w365 -> [w367]
                  stop <- w369 stop-if-true
                  n85 = call "Elapsed Time"("Time Target (s)"=w367) -> ("Elapsed Time (s)"=w368:dbl, "Time has Elapsed"=w369:bool)  [unwired: 11 in, 6 out]
                  n86 = Subtract(x=w367, y=w368) -> (x-y=→"Time until next cycle":dbl)
                }
              }
              frame True {
              }
            }
            n87 = stacked-sequence {
              frame #0 {
                n88 = property on="CAEN 1.0" class="Knob (strict)"("Scale.Minimum"="Scale.Range:Minimum", "Scale.Maximum"="Scale.Range:Maximum") -> ()  [unwired: 2 in, 2 out]
                n89 = property on="CAEN 1.1" class="Knob (strict)"("Scale.Minimum"="Scale.Range:Minimum 2", "Scale.Maximum"="Scale.Range:Maximum 2") -> ()  [unwired: 2 in, 2 out]
              }
              frame #1 {
                n90 = property on="CAEN 1.2" class="Knob (strict)"("Scale.Minimum"="Scale.Range:Minimum 3", "Scale.Maximum"="Scale.Range:Maximum 3") -> ()  [unwired: 2 in, 2 out]
                n91 = property on="CAEN 1.3" class="Knob (strict)"("Scale.Maximum"="Scale.Range:Maximum 4", "Scale.Minimum"="Scale.Range:Minimum 4") -> ()  [unwired: 2 in, 2 out]
              }
              frame #2 {
                n92 = property on="CAEN 2.1" class="Knob (strict)"("Scale.Maximum"="Scale.Range:Maximum 6", "Scale.Minimum"="Scale.Range:Minimum 6") -> ()  [unwired: 2 in, 2 out]
                n93 = property on="CAEN 2.0" class="Knob (strict)"("Scale.Maximum"="Scale.Range:Maximum 5", "Scale.Minimum"="Scale.Range:Minimum 5") -> ()  [unwired: 2 in, 2 out]
              }
              frame #3 {
                n94 = property on="CAEN 2.2" class="Knob (strict)"("Scale.Maximum"="Scale.Range:Maximum 7", "Scale.Minimum"="Scale.Range:Minimum 7") -> ()  [unwired: 2 in, 2 out]
                n95 = property on="CAEN 2.3" class="Knob (strict)"("Scale.Maximum"="Scale.Range:Maximum 8", "Scale.Minimum"="Scale.Range:Minimum 8") -> ()  [unwired: 2 in, 2 out]
              }
            }
          }
          frame #1 {
            # "DAQmx Read above will replace dummy data below,\nonce the 9216 modules are functioning"
            # "Descr"
            # "NI 9207 8x V, 8x mA"
            # "Case to ignore runtime errors; unpack later"
            # "Module 1 tasks+status"
            # "Temps (NI)"
            # "9216 T     (NI) x16\n9207 V     (NI)  x8\n9207 mA (NI)  x8\nTemp        (LS)  x2\nHeater %           x1"
            # "Temp A, Temp B, heater power"
            # "Measurements and conversions"
            n96 = case shown="True" "Run lakeshore?" {
              tunnel: [w436 w447] -> w413
              tunnel: w412 -> [w436 w446]
              tunnel: [-273.0 ("Input A") w445] -> w409
              tunnel: [-273.0 ("Input B") w444] -> w408
              tunnel: [73.0 ("Heater 1 (%)") w443] -> w407
              tunnel: w406 -> [_ w441]
              tunnel: [-274.0 "Setpoint (°C)"] -> w403
              frame False {
                # "Dummy data"
              }
              frame True {
                # "LS output"
                # "P\nI\nD"
                n97 = Select(t=0, s=w441, f="Heater range") -> (s? t:f=w438:i32)
                n98 = Unbundle("PID settings") -> ("P"=w452:dbl, "I"=w451:dbl, "D"=w450:dbl)
                n99 = Unbundle(w446) -> ("VISA resource name out"=w454:refnum<visa-resource-name>, "error out"=w453:errorcluster)
                n100 = call "Lakeshore subVI.vi"("Setpoint"="Setpoint (°C)", "Rate (D) (X.X %)"=w450, "Range"=w438, "Reset (I) (XX.X)"=w451, "Gain (P) (XX.X)"=w452, "error in (no error)"=w453, "VISA resource name"=w454) -> ("Input B"=w444:dbl, "Input A"=w445:dbl, "error out"=w448:errorcluster, "VISA resource name out"=w449:refnum<visa-resource-name>, "Heater 1 (%)"=w443:dbl)
                "Lakeshore" <- w448
                n101 = Bundle("VISA resource name out"=w449, "error out"=w448) -> (w447:T5)  [unwired: 1 in]
              }
            }
            n102 = Get Date/Time In Seconds() -> (seconds since 1Jan1904=w411:timestamp)
            n103 = Quotient & Remainder(x=w399, y="Read T every N cycles") -> (x-y*floor(x/y)=w402:i32)  [unwired: 1 out]
            n104 = Unbundle(w385) -> ("task out"=w384:refnum<k21>, "error out"=w383:errorcluster)
            n105 = Build Array (concatenate)(w378, w411) -> (w410:timestamp[])
            n106 = Unbundle(w405) -> ("task out"=w390:refnum<k21>, "error out"=w389:errorcluster)
            n107 = case shown="1, Default" w402 {
              tunnel: w400 -> [_ w429]
              tunnel: [w422 w425] -> w370
              tunnel: w399 -> [w421 _]
              frame 0 {
                # "Dummy data"
                # "New temperatures"
                n108 = Add(x=w421, y=-95.0 ("element")) -> (x+y=w424:dbl)
                n109 = Initialize Array(w424, 16) -> (w422:dbl[])
              }
              frame 1, Default {
                # "Gets 1st 16 Col's\nfrom last row:\nPrevious 16 temps."
                # "Get previous temps"
                n110 = Array Size(array=w429) -> (size(s)=w431:i32[])
                n111 = Index Array(array=w431, index=0) -> (element=w432:i32)
                n112 = Decrement(x=w432) -> (x-1=w428:i32)
                n113 = Index Array(array=w429, index (row)=w428) -> (element=w427:dbl[])  [unwired: 1 in]
                n114 = Array Subset(array=w427, length=16) -> (w425:dbl[])  [unwired: 1 in]
              }
            }
            n115 = call-poly <vilib>:"DAQmx Read.vi"("task/channels in"=w384, "error in"=w383) -> ("task out"=w382:refnum<k21>, "data"=→"PT100 data":dbl[], "error out"=w381:errorcluster)  [unwired: 11 in]
            "NI 9216 x2" <- w381
            n116 = call-poly <vilib>:"DAQmx Read.vi"("task/channels in"=w390, "error in"=w389) -> ("task out"=w388:refnum<k21>, "data"=w397:dbl[], "error out"=w387:errorcluster)  [unwired: 11 in]
            "Raw readouts (V, mA)" <- w397
            "NI 9207" <- w387
            n117 = Build Array (concatenate)("Offsets\nsubtracted", "Offsets\nsubtracted") -> (w391:dbl[])
            n118 = Build Array (concatenate)("Multipliers", "Multipliers") -> (w394:dbl[])
            n119 = for {
              tunnel: w391 -> [w419] mode=indexing
              tunnel: w397 -> [w418] mode=indexing
              tunnel: w394 -> [w416] mode=indexing
              tunnel: [w415] -> w398 mode=indexing
              n120 = Subtract(x=w418, y=w419) -> (x-y=w417:dbl)
              n121 = Multiply(x=w417, y=w416) -> (x*y=w415:dbl)
            }
            n122 = Bundle("task out"=w382, "error out"=w381) -> (w380:T4)  [unwired: 1 in]
            n123 = Bundle("task out"=w388, "error out"=w387) -> (w401:T4)  [unwired: 1 in]
            n124 = Build Array(w409, w408, w407) -> (w386:dbl[])
            "LakeShore readings" <- w386
            n125 = Unbundle(w377) -> ("task out"=w376:refnum<k21>, "error out"=w375:errorcluster)
            n126 = call-poly <vilib>:"DAQmx Read.vi"("task/channels in"=w376, "error in"=w375) -> ("task out"=w374:refnum<k21>, "data"=w371:dbl[], "error out"=w373:errorcluster)  [unwired: 11 in]
            "NI 9226" <- w373
            "PT1000 data" <- w371
            n127 = Bundle("task out"=w374, "error out"=w373) -> (w372:T4)  [unwired: 1 in]
          }
          frame #2 {
            # "Alter voltages if button clicked"
            # "2"
            # "1"
            # "Descr."
            # "Descr."
            # "VMON1  x4 \nVMON2  x4\nIMON1    x4\nIMON2    x4"
            # "Needle gauge Voltage displays"
            # "1"
            # "2"
            # "1"
            # "2"
            # "Reads new V and A every N cycles,\nor passes previous values"
            # "High Voltage"
            n128 = Quotient & Remainder(x=w493, y="Read CAEN units \nevery N cycles") -> (x-y*floor(x/y)=w472:i32)  [unwired: 1 out]
            n129 = Unbundle(w500) -> ("VISA resource name out"=w464:refnum<visa-resource-name>, "error out"=w499:errorcluster)
            n130 = Unbundle(w497) -> ("VISA resource name out"=w463:refnum<visa-resource-name>, "error out"=w496:errorcluster)
            n131 = Build Array (concatenate)("VSet (V)", "VMax (V)", "IMax (uA)") -> (w477:dbl[])
            n132 = case shown="0" w472 {
              tunnel: w464 -> [w641 _]
              tunnel: w499 -> [w640 w652]
              tunnel: w498 -> [_ w648]
              tunnel: w463 -> [w634 _]
              tunnel: w496 -> [w631 w653]
              tunnel: [w630 w653] -> w458
              tunnel: [w637 w652] -> w461
              tunnel: [w623 w648] -> w468
              tunnel: [w625 w649] -> w495
              tunnel: [w624 w645] -> w494
              tunnel: w462 -> [w626 _]
              frame 0 {
                # "All data x16"
                # "Voltages x8"
                # "Currents x8"
                # "Read"
                n133 = call "READ_SUPPLY.vi"("VISA resource name"=w641, "Board address"=u8 0, "NChannels"=u8 4, "error in (no error)"=w640) -> ("VMon values (V)"=w636:dbl[], "IMon values (uA)"=w635:dbl[], "error out"=w637:errorcluster)  [unwired: 9 in]
                n134 = call "READ_SUPPLY.vi"("VISA resource name"=w634, "Board address"=u8 0, "NChannels"=u8 4, "error in (no error)"=w631) -> ("VMon values (V)"=w629:dbl[], "IMon values (uA)"=w628:dbl[], "error out"=w630:errorcluster)  [unwired: 9 in]
                n135 = Build Array (concatenate)(w636, w629) -> (w627:dbl[])
                n136 = Build Array (concatenate)(w635, w628) -> (w624:dbl[])
                n137 = for {
                  tunnel: w627 -> [w643] mode=indexing
                  tunnel: w626 -> [w644] mode=indexing
                  tunnel: [w642] -> w625 mode=indexing
                  n138 = Multiply(x=w644, y=w643) -> (x*y=w642:dbl)
                }
                n139 = Build Array (concatenate)(w625, w624) -> (w623:dbl[])
              }
              frame 1, Default {
                # "Don't read: pass previous"
                n140 = Array Subset(array=w648, index=0, length=8) -> (w649:dbl[])
                n141 = Array Subset(array=w648, index=8, length=8) -> (w645:dbl[])
              }
            }
            "Voltages" <- w495
            "Vmon (V)" <- w495
            "IMon (uA)" <- w494
            n142 = Build Array("Apply Voltage", "Set to zero", "Kill voltage") -> (w471:bool[])
            n143 = case shown="True" "Query HV status" {
              tunnel: w464 -> [_ w512]
              tunnel: w463 -> [_ w511]
              tunnel: w458 -> [w501 w506]
              tunnel: w461 -> [w502 w505]
              tunnel: [w502 w504] -> w466
              tunnel: [w501 w503] -> w465
              frame False {
              }
              frame True {
                w514 = u8 0 ("Board address")
                w513 = u8 4 ("NChannels")
                n144 = Bundle("VISA resource name out"=w512, "Board address"=w514, "NChannels"=w513) -> (w509:T6)  [unwired: 1 in]
                n145 = Bundle("VISA resource name out"=w511, "Board address"=w514, "NChannels"=w513) -> (w510:T6)  [unwired: 1 in]
                n146 = call <instrlib>:"Channel Status.vi"("error in (no error)"=w505, "BoardHandle"=w509) -> ("error out"=w504:errorcluster, "Channel Status Array"=→"CAEN 1":T2)  [unwired: 7 in, 1 out]
                n147 = call <instrlib>:"Channel Status.vi"("error in (no error)"=w506, "BoardHandle"=w510) -> ("error out"=w503:errorcluster, "Channel Status Array"=→"CAEN 2":T2)  [unwired: 7 in, 1 out]
              }
            }
            n148 = Search 1D Array(1D array=w471, element=TRUE) -> (index of element=w485:i32)  [unwired: 1 in]
            n149 = case shown="0" w485 {
              tunnel: w464 -> [w528 w563 w596 w622]
              tunnel: w463 -> [w518 w555 w587 w621]
              tunnel: [w529 w564 w597 w620] -> w460
              tunnel: [w528 w563 w596 w622] -> w484
              tunnel: [w517 w554 w586 w619] -> w457
              tunnel: [w518 w555 w587 w621] -> w482
              tunnel: "VSet (V)" -> [w526 _ w594 _]
              tunnel: "VMax (V)" -> [w525 w561 _ _]
              tunnel: "IMax (uA)" -> [w524 w560 w593 _]
              tunnel: w466 -> [w516 w553 w585 w620]
              tunnel: w465 -> [w515 w552 w584 w619]
              frame 0 {
                w519 = 4 ("length")
                w523 = 4 ("length")
                # "Last four"
                # "First four"
                # "Apply voltage"
                n150 = Array Subset(array=w526, length=w523) -> (w531:dbl[])  [unwired: 1 in]
                n151 = Array Subset(array=w525, length=w523) -> (w530:dbl[])  [unwired: 1 in]
                n152 = Array Subset(array=w524, length=w523) -> (w527:dbl[])  [unwired: 1 in]
                n153 = Array Subset(array=w526, index=w519) -> (w522:dbl[])  [unwired: 1 in]
                n154 = Array Subset(array=w525, index=w519) -> (w521:dbl[])  [unwired: 1 in]
                n155 = Array Subset(array=w524, index=w519) -> (w520:dbl[])  [unwired: 1 in]
                n156 = for {
                  tunnel: w528 -> [w550]
                  tunnel: w516 -> [w549]
                  tunnel: w531 -> [w546] mode=indexing
                  tunnel: w530 -> [w544] mode=indexing
                  tunnel: w527 -> [w543] mode=indexing
                  tunnel: [w542] -> w529
                  i -> [w551]
                  n157 = call "SET_SUPPLY_CHANNEL.vi"("VISA resource name"=w550, "Voltage Level (0.0 V)"=w546, "Enable (OFF)"=TRUE, "Board address"=u8 0, "NChannels"=u8 4, "Channel (0)"=w551, "error in (no error)"=w549, "Voltage Max (0.0 V)"=w544, "Current Limit (0.00 uA)"=w543) -> ("error out"=w542:errorcluster)  [unwired: 6 in]
                }
                n158 = for {
                  tunnel: w518 -> [w541]
                  tunnel: w515 -> [w535]
                  tunnel: w522 -> [w540] mode=indexing
                  tunnel: w521 -> [w539] mode=indexing
                  tunnel: w520 -> [w538] mode=indexing
                  tunnel: [w534] -> w517
                  i -> [w537]
                  n159 = call "SET_SUPPLY_CHANNEL.vi"("VISA resource name"=w541, "Voltage Level (0.0 V)"=w540, "Enable (OFF)"=TRUE, "Board address"=u8 0, "NChannels"=u8 4, "Channel (0)"=w537, "error in (no error)"=w535, "Voltage Max (0.0 V)"=w539, "Current Limit (0.00 uA)"=w538) -> ("error out"=w534:errorcluster)  [unwired: 6 in]
                }
              }
              frame 1 {
                w556 = 4 ("length")
                w559 = 4 ("length")
                # "Set V to zero"
                n160 = Array Subset(array=w560, length=w559) -> (w562:dbl[])  [unwired: 1 in]
                n161 = Array Subset(array=w561, length=w559) -> (w565:dbl[])  [unwired: 1 in]
                n162 = Array Subset(array=w561, index=w556) -> (w558:dbl[])  [unwired: 1 in]
                n163 = Array Subset(array=w560, index=w556) -> (w557:dbl[])  [unwired: 1 in]
                n164 = for {
                  tunnel: w563 -> [w582]
                  tunnel: w553 -> [w581]
                  tunnel: w565 -> [w578] mode=indexing
                  tunnel: w562 -> [w577] mode=indexing
                  tunnel: [w576] -> w564
                  i -> [w583]
                  w575 = u8 0 ("Board address")
                  n165 = call "SET_SUPPLY_CHANNEL.vi"("VISA resource name"=w582, "Voltage Level (0.0 V)"=w575, "Enable (OFF)"=TRUE, "Board address"=w575, "NChannels"=u8 4, "Channel (0)"=w583, "error in (no error)"=w581, "Voltage Max (0.0 V)"=w578, "Current Limit (0.00 uA)"=w577) -> ("error out"=w576:errorcluster)  [unwired: 6 in]
                }
                n166 = for {
                  tunnel: w555 -> [w566]
                  tunnel: w552 -> [w571]
                  tunnel: w558 -> [w570] mode=indexing
                  tunnel: w557 -> [w569] mode=indexing
                  tunnel: [w567] -> w554
                  i -> [w572]
                  w574 = 0 ("length")
                  n167 = call "SET_SUPPLY_CHANNEL.vi"("VISA resource name"=w566, "Voltage Level (0.0 V)"=w574, "Enable (OFF)"=TRUE, "Board address"=w574, "NChannels"=u8 4, "Channel (0)"=w572, "error in (no error)"=w571, "Voltage Max (0.0 V)"=w570, "Current Limit (0.00 uA)"=w569) -> ("error out"=w567:errorcluster)  [unwired: 6 in]
                }
              }
              frame 2 {
                w588 = 4 ("length")
                w591 = 2 ("length")
                w592 = 4 ("length")
                # "CAEN 2: Top gate, Bottom gate"
                # "CAEN 1 values:\nPMT1&2, Anode, Cathode"
                # "Set VMax to zero, \"Kill\""
                n168 = Array Subset(array=w593, length=w592) -> (w595:dbl[])  [unwired: 1 in]
                n169 = Array Subset(array=w594, length=w592) -> (w598:dbl[])  [unwired: 1 in]
                n170 = Array Subset(array=w594, index=w588, length=w591) -> (w590:dbl[])
                n171 = Array Subset(array=w593, index=w588, length=w591) -> (w589:dbl[])
                n172 = for {
                  tunnel: w596 -> [w617]
                  tunnel: w585 -> [w616]
                  tunnel: w598 -> [w613] mode=indexing
                  tunnel: w595 -> [w611] mode=indexing
                  tunnel: [w610] -> w597
                  i -> [w618]
                  n173 = call "SET_SUPPLY_CHANNEL.vi"("VISA resource name"=w617, "Voltage Level (0.0 V)"=w613, "Enable (OFF)"=TRUE, "Board address"=u8 0, "NChannels"=u8 4, "Channel (0)"=w618, "error in (no error)"=w616, "Voltage Max (0.0 V)"=u8 0 ("Board address"), "Current Limit (0.00 uA)"=w611) -> ("error out"=w610:errorcluster)  [unwired: 6 in]
                }
                n174 = for {
                  tunnel: w587 -> [w599]
                  tunnel: w584 -> [w602]
                  tunnel: w590 -> [w605] mode=indexing
                  tunnel: w589 -> [w603] mode=indexing
                  tunnel: [w601] -> w586
                  i -> [w608]
                  n175 = call "SET_SUPPLY_CHANNEL.vi"("VISA resource name"=w599, "Voltage Level (0.0 V)"=w605, "Enable (OFF)"=TRUE, "Board address"=u8 0, "NChannels"=u8 4, "Channel (0)"=w608, "error in (no error)"=w602, "Voltage Max (0.0 V)"=0, "Current Limit (0.00 uA)"=w603) -> ("error out"=w601:errorcluster)  [unwired: 6 in]
                }
              }
              frame 3, Default {
                # "\"Executes\" if none of the three buttons have been clicked"
                # "Do nothing"
              }
            }
            n176 = Merge Errors(w461, w460) -> (→"CAEN 1":errorcluster)
            n177 = Bundle("VISA resource name out"=w484, "error out"=w460) -> (w483:T5)  [unwired: 1 in]
            n178 = Bundle("VISA resource name out"=w482, "error out"=w457) -> (w481:T5)  [unwired: 1 in]
            n179 = Merge Errors(w458, w457) -> (→"CAEN 2":errorcluster)
            n180 = Index Array(array=w468) -> (element #1=→"CAEN 1.0":dbl, element #2=→"CAEN 1.1":dbl, element #3=→"CAEN 1.2":dbl, element #4=→"CAEN 1.3":dbl, element #5=→"CAEN 2.0":dbl, element #6=→"CAEN 2.1":dbl, element #7=→"CAEN 2.2":dbl, element #8=→"CAEN 2.3":dbl)  [unwired: 8 in]
          }
          frame #3 {
            # "Descr."
            # "Reset anode"
            n181 = Or Array Elements(Boolean array=w655) -> (logical OR=w654:bool)
            n182 = case shown="True" "Reset anode\nperiodically?" {
              tunnel: w662 -> [_ w668]
              tunnel: w661 -> [_ w677]
              tunnel: w660 -> [_ w682]
              tunnel: w654 -> [_ w666]
              tunnel: [w663 w667] -> w657
              tunnel: w656 -> [_ w676]
              frame False {
                # "Anode Reset Routine inactive:\nkeep timers up to date so activating\nroutine will correctly initiate the timers."
                n183 = Get Date/Time In Seconds() -> (seconds since 1Jan1904=w665:timestamp)
                n184 = To Double Precision Float(number=w665) -> (double precision float=w664:dbl)
                n185 = Build Array(w664, w664) -> (w663:dbl[])
              }
              frame True {
                # "Descr."
                n186 = case shown="\"CAEN 1\", Default" "CAEN unit selector" {
                  tunnel: w677 -> [w696 _]
                  tunnel: w676 -> [_ w698]
                  tunnel: [w696 w698] -> w675
                  tunnel: [0 4] -> w673
                  frame "CAEN 1", Default {
                  }
                  frame "CAEN 2" {
                  }
                }
                n187 = call "anode_timing.vi"("Keep off for X seconds"="Keep off for X seconds", "Array of timers"=w668, "Kill every Y minutes"="Kill every Y minutes") -> ("Time to kill"=w684:bool, "Time until reset"=→"Seconds until \nanode reset":dbl, "Time until autokill"=→"Seconds until \nanode autokill":dbl, "Time to reset"=w685:bool)  [unwired: 5 in]
                "Killed" <- w684
                "Restarted" <- w685
                n188 = Add(x=w673, y="Anode ch.") -> (x+y=w671:i32)
                n189 = Build Array(w684, w685, w666) -> (w688:bool[])
                n190 = Add(x=w671, y=8) -> (x+y=w678:i32)
                n191 = Add(x=w671, y=16) -> (x+y=w679:i32)
                n192 = Search 1D Array(1D array=w688, element=TRUE) -> (index of element=w687:i32)  [unwired: 1 in]
                n193 = Unbundle(w675) -> ("VISA resource name out"=w693:refnum<visa-resource-name>, "error out"=w692:errorcluster)
                n194 = Index Array(array=w682, index #1=w671, index #2=w678, index #3=w679) -> (element #1=w691:dbl, element #2=w689:dbl, element #3=w690:dbl)
                n195 = case shown="2" w687 {
                  tunnel: w691 -> [_ w722 _ _]
                  tunnel: w689 -> [w707 w721 _ _]
                  tunnel: w690 -> [w709 w720 _ _]
                  tunnel: w693 -> [w714 w725 _ _]
                  tunnel: w692 -> [w713 w724 _ _]
                  tunnel: "Anode ch." -> [w705 w718 _ _]
                  tunnel: w668 -> [w700 _ _ w731]
                  tunnel: [w699 w715 w728 w731] -> w667
                  frame 0 {
                    # "Set Anode Voltage to zero,\nreset the 1st timer"
                    # "Anode Vset to zero"
                    n196 = Get Date/Time In Seconds() -> (seconds since 1Jan1904=w703:timestamp)
                    n197 = Index Array(array=w700, index=1) -> (element=w701:dbl)
                    n198 = To Double Precision Float(number=w703) -> (double precision float=w702:dbl)
                    n199 = call "SET_SUPPLY_CHANNEL.vi"("VISA resource name"=w714, "Voltage Level (0.0 V)"=0.0, "Enable (OFF)"=TRUE, "Board address"=u8 0, "NChannels"=u8 4, "Channel (0)"=w705, "error in (no error)"=w713, "Voltage Max (0.0 V)"=w707, "Current Limit (0.00 uA)"=w709) -> ("error out"=w708:errorcluster)  [unwired: 6 in]
                    n200 = Build Array(w702, w701) -> (w699:dbl[])
                    n201 = call <vilib>:"Simple Error Handler.vi"("error in (no error)"=w708) -> ()  [unwired: 4 in, 5 out]
                  }
                  frame 1 {
                    # "Set Anode Voltage to defined value,\nreset both timers"
                    # "Anode Vset applied"
                    n202 = Get Date/Time In Seconds() -> (seconds since 1Jan1904=w717:timestamp)
                    n203 = To Double Precision Float(number=w717) -> (double precision float=w716:dbl)
                    n204 = call "SET_SUPPLY_CHANNEL.vi"("VISA resource name"=w725, "Voltage Level (0.0 V)"=w722, "Enable (OFF)"=TRUE, "Board address"=u8 0, "NChannels"=u8 4, "Channel (0)"=w718, "error in (no error)"=w724, "Voltage Max (0.0 V)"=w721, "Current Limit (0.00 uA)"=w720) -> ("error out"=w719:errorcluster)  [unwired: 6 in]
                    n205 = Build Array(w716, w716) -> (w715:dbl[])
                    n206 = call <vilib>:"Simple Error Handler.vi"("error in (no error)"=w719) -> ()  [unwired: 4 in, 5 out]
                  }
                  frame 2 {
                    # "Change Voltage button pressed"
                    # "Reset both timers"
                    n207 = Get Date/Time In Seconds() -> (seconds since 1Jan1904=w730:timestamp)
                    n208 = To Double Precision Float(number=w730) -> (double precision float=w729:dbl)
                    n209 = Build Array(w729, w729) -> (w728:dbl[])
                  }
                  frame 3, Default {
                    # "Timers stay at previous value,\nso difference between those and\ncurrent time keeps incrementing"
                    # "No event"
                  }
                }
              }
            }
            n210 = To Time Stamp(1:w657) -> (0:→"Anode timers":timestamp[])
            "?" <- "Reset anode\nperiodically?"
          }
          frame #4 {
            # "Det. P"
            # "Flow"
            # "Flexibly acquire indices"
            # "Plots 9207 output vs time"
            # "Descr."
            # "Moving averages"
            # "Historic graphs: Phase, 9207 ai, Flow, Heater, Temperature"
            # "Non-historic Temperature + Det. Pressure"
            # "Updated TOBA"
            # "Descr."
            # "Latest Detector Pressure"
            # "Plots individual lists of Temp. vs. t"
            # "Plots and moving averages"
            n211 = Build Array (concatenate)(w750, w733, w747, w749) -> (w778:dbl[])
            n212 = Build Array (concatenate)(w779, w778) -> (w736:dbl[][])
            "TOBA appended" <- w736
            n213 = Array Size(array=w747) -> (size(s)=w746:i32)
            n214 = Array Size(array=w733) -> (size(s)=w748:i32)
            n215 = Array Size(array=w750) -> (size(s)=w734:i32)
            n216 = Add(x=w734, y=w748) -> (x+y=w739:i32)
            n217 = Add(x=w739, y=w746) -> (x+y=w745:i32)
            n218 = local read "Flow input #"() -> (w756:i32)
            n219 = local read "Det.P input #"() -> (w757:i32)
            n220 = Add(x=w745, y=2 ("disabled index (col)")) -> (x+y=w743:i32)
            n221 = Equal?(x=666, y="Temperature channel selector") -> (x = y?=w772:bool)
            n222 = Index Array(array=w736, index (col)=w743) -> (element=w742:dbl[])  [unwired: 1 in]
            n223 = case shown="True" w772 {
              tunnel: w733 -> [w817 w818]
              tunnel: [w816 w819] -> w770
              tunnel: "Temperature channel selector" -> [w815 _]
              frame False {
                n224 = Index Array(array=w817, index=w815) -> (element=w816:dbl)
              }
              frame True {
                n225 = Add Array Elements(numeric array=w818) -> (sum=w820:dbl)
                n226 = Array Size(array=w818) -> (size(s)=w821:i32)
                n227 = Divide(x=w820, y=w821) -> (x/y=w819:dbl)
              }
            }
            n228 = Add(x=w757, y=w739) -> (x+y=w766:i32)
            n229 = Add(x=w739, y=w756) -> (x+y=w764:i32)
            n230 = Bundle(w735, w742) -> (w738:cluster{timestamp[], dbl[]})  [unwired: 1 in]
            n231 = Build Array(w738) -> (→"Heater power (%)":cluster{timestamp[], dbl[]}[])
            n232 = Add(x=w734, y="Temperature Channel Selector") -> (x+y=w740:i32)
            n233 = Index Array(array=w736, index (col) #1=w766, index (col) #2=w764) -> (element #1=w765:dbl[], element #2=w754:dbl[])  [unwired: 2 in]
            n234 = local read "Det.P input #"() -> (w758:i32)
            n235 = Index Array(array=w736, index (col)=w740) -> (element=w769:dbl[])  [unwired: 1 in]
            n236 = for {
              N: 8 -> [_]
              tunnel: w736 -> [w808]
              tunnel: w735 -> [w801]
              tunnel: [w805] -> w762 mode=indexing
              tunnel: [w800] -> w761 mode=indexing
              tunnel: w739 -> [w798]
              i -> [w804]
              n237 = Add(x=w798, y=8) -> (x+y=w797:i32)
              n238 = Add(x=w798, y=w804) -> (x+y=w807:i32)
              n239 = Add(x=w804, y=w797) -> (x+y=w803:i32)
              n240 = Index Array(array=w808, index (col) #1=w807, index (col) #2=w803) -> (element #1=w806:dbl[], element #2=w802:dbl[])  [unwired: 2 in]
              n241 = Bundle(w801, w806) -> (w805:cluster{timestamp[], dbl[]})  [unwired: 1 in]
              n242 = Bundle(w801, w802) -> (w800:cluster{timestamp[], dbl[]})  [unwired: 1 in]
            }
            "9207 (ai 0:7, Volts)" <- w762
            "9207 (ai 8:15, Amperes)" <- w761
            n243 = Bundle(w769, w765) -> (w783:cluster{dbl[], dbl[]})  [unwired: 1 in]
            n244 = Index Array(array=w747, index=w758) -> (element=w784:dbl)
            n245 = Bundle(w735, w754) -> (w781:cluster{timestamp[], dbl[]})  [unwired: 1 in]
            n246 = Build Array(w783) -> (→"Historical Large Phase Diagram":cluster{dbl[], dbl[]}[])
            n247 = Bundle("Waveform"=w770, w784) -> (w788:cluster{"Waveform":dbl, dbl})  [unwired: 1 in]
            n248 = Build Array(w781) -> (→"Flow (SLPM)":cluster{timestamp[], dbl[]}[])
            n249 = call "moving_avg.vi"("N samples"="N samples", "Array"=w765) -> ("Numeric"=→"Detector Pressure":dbl)  [unwired: 9 in]
            n250 = call "moving_avg.vi"("N samples"="N samples", "Array"=w754) -> ("Numeric"=→"Average Flow (SLPM)":dbl)  [unwired: 9 in]
            n251 = Build Array(w788) -> (→"Phase Diagram":cluster{"Waveform":dbl, dbl}[])
            n252 = for {
              N: w734 -> [_]
              tunnel: w735 -> [w833]
              tunnel: [w832] -> w789 mode=indexing
              tunnel: w736 -> [w831]
              i -> [w829]
              n253 = Index Array(array=w831, index (col)=w829) -> (element=w830:dbl[])  [unwired: 1 in]
              n254 = Bundle(w833, w830) -> (w832:cluster{timestamp[], dbl[]})  [unwired: 1 in]
            }
            "Temperature (9216 0:15, °C)" <- w789
            n255 = Array Size(array=w733) -> (size(s)=w732:i32)
            n256 = Equal?(x=666, y="Temperature Channel Selector") -> (x = y?=w774:bool)
            n257 = local read "Channel Names (9207, ai0:7)"() -> (w759:string[])
            n258 = local read "Channel Names (9207, ai8:15)"() -> (w760:string[])
            n259 = case shown="False" w774 {
              tunnel: w733 -> [w824 w825]
              tunnel: [w823 w826] -> w777
              tunnel: "Temperature Channel Selector" -> [w822 _]
              frame False {
                n260 = Index Array(array=w824, index=w822) -> (element=w823:dbl)
              }
              frame True {
                n261 = Add Array Elements(numeric array=w825) -> (sum=w827:dbl)
                n262 = Array Size(array=w825) -> (size(s)=w828:i32)
                n263 = Divide(x=w827, y=w828) -> (x/y=w826:dbl)
              }
            }
            n264 = for {
              N: w732 -> [_]
              tunnel: w735 -> [w796]
              tunnel: [w795] -> _ mode=indexing
              tunnel: w736 -> [w794]
              tunnel: w734 -> [w790]
              i -> [w791]
              n265 = Add(x=w790, y=w791) -> (x+y=w792:i32)
              n266 = Index Array(array=w794, index (col)=w792) -> (element=w793:dbl[])  [unwired: 1 in]
              n267 = Bundle(w796, w793) -> (w795:cluster{timestamp[], dbl[]})  [unwired: 1 in]
            }
            n268 = call "Is Value Changed.vim"("value"=w760) -> ("changed or first call?"=w767:bool)
            n269 = call "Is Value Changed.vim"("value"=w759) -> ("changed or first call?"=w768:bool)
            n270 = case shown="True" w767 {
              tunnel: w760 -> [_ w809]
              frame False {
              }
              frame True {
                n271 = for {
                  tunnel: w809 -> [w810] mode=indexing
                  i -> [w811]
                  n272 = property on="9207 (ai 8:15, Amperes)" class="XYGraph (strict)"("Active Plot"=w811, "Plot.Plot Name"=w810) -> ()  [unwired: 2 in, 2 out]
                }
              }
            }
            n273 = case shown="True" w768 {
              tunnel: w759 -> [_ w812]
              frame False {
              }
              frame True {
                n274 = for {
                  tunnel: w812 -> [w813] mode=indexing
                  i -> [w814]
                  n275 = property on="9207 (ai 0:7, Volts)" class="XYGraph (strict)"("Active Plot"=w814, "Plot.Plot Name"=w813) -> ()  [unwired: 2 in, 2 out]
                }
              }
            }
            n276 = Bundle("Waveform"=w777, w784) -> (w786:cluster{"Waveform":dbl, dbl})  [unwired: 1 in]
            n277 = Build Array(w786) -> (→"Large Phase Diagram":cluster{"Waveform":dbl, dbl}[])
          }
          frame #5 {
            # "Temp A, Temp B, Heater%"
            # "Temperatures x16\nTo indicators on the physical schematic"
            # "Individual latest 9207 readings.\nIndicators go here. Array is 1x16,\nitems have been converted using\nthe offsets and multipliers"
            # "Displays"
            n278 = local read "Flow input #"() -> (w837:i32)
            n279 = case shown="False" "Reset?" {
              tunnel: [w849 0.0] -> w845
              tunnel: w842 -> [w849 _]
              frame False {
              }
              frame True {
              }
            }
            n280 = Index Array(array=w836) -> ()  [unwired: 16 in, 16 out]
            n281 = Index Array(array=w836, index=w837) -> (element=w840:dbl)
            n282 = call "Average_flow_x_time.vi"("Array of timestamps"=w844, "Previous Flow"=w843, "Latest Flow"=w840) -> ("Volume (SL)"=w846:dbl)  [unwired: 8 in]
            n283 = case shown="False" "Pause?" {
              tunnel: w845 -> [w853 w854]
              tunnel: w846 -> [w852 _]
              tunnel: [w851 w854] -> w841
              frame False {
                n284 = Add(x=w852, y=w853) -> (x+y=w851:dbl)
              }
              frame True {
              }
            }
            "Integrated Flow (SL)" <- w841
            n285 = Index Array(array=w838) -> (element #1=→"Coldhead" →"Temp A":dbl, element #2=→"Heater" →"Temp B":dbl)  [unwired: 3 in, 1 out]
            n286 = Index Array(array=w839) -> ()  [unwired: 16 in, 16 out]
            "9207 (V; A) Converted" <- w836
            "9216 #1 (°C)" <- w839
            "9216 #2 (°C)" <- w839
          }
          frame #6 {
            # "9226 not being saved rn"
            # "The same order applies to the headers re-saved,\nbut with an additional line, stating the date/time"
            # "-----------DATA SAVED----------\nHuman-readable timestamp  ;\nTemperatures (16),  2xNI 9216;\nVolts, Amps  (8 x2),     NI 9207;\nTemperature (2),    Lakeshore;\nHeater power (1),  Lakeshore;\nSetpoint (1),           Lakeshore;\nHV readouts (16)          CAEN ;\nCurrent time (s)                ---   ;\nCycle time (s)                    ---   ;"
            # "Saving data"
            n287 = Get Date/Time In Seconds() -> (seconds since 1Jan1904=w876:timestamp)
            n288 = To Double Precision Float(number=w876) -> (double precision float=w862:dbl)
            n289 = Build Array (concatenate)(w857, w865, w864, w877, w863, w862, w861) -> (w875:dbl[])
            n290 = Array Size(array=w857) -> (size(s)=w858:i32)
            n291 = Array Size(array=w856) -> (size(s)=w859:i32)
            n292 = Add(x=w858, y=w859) -> (x+y=w855:i32)
            n293 = Get Date/Time String() -> (date string=w869:string)  [unwired: 3 in, 1 out]
            n294 = case shown="True" "Re-save headers" {
              tunnel: w855 -> [_ w878]
              frame False {
                # "Just sit around and feel pretty"
              }
              frame True {
                w886 = ""
                # "Append line of most recent channel names to header file"
                n295 = local read "Channel Names (CAEN)"() -> (w885:string[])
                n296 = local read "Channel Names (9207, ai0:7)"() -> (w893:string[])
                n297 = for {
                  N: w878 -> [_]
                  shift-right: [w917] -> w889
                  shift-left: "" -> [w918]
                  i -> [w922]
                  n298 = Format Into String(initial string="t", w922) -> (resulting string=w920:string)  [unwired: 2 in, 1 out]
                  n299 = Concatenate Strings(w918, w920, "\t") -> (w917:string)
                }
                n300 = for {
                  shift-right: [w915] -> w891
                  shift-left: w886 -> [w916]
                  tunnel: w893 -> [w913] mode=indexing
                  n301 = Concatenate Strings(w916, w913, "\t") -> (w915:string)
                }
                n302 = local read "Channel Names (9207, ai8:15)"() -> (w892:string[])
                n303 = for {
                  tunnel: w885 -> [w907] mode=indexing
                  shift-right: [w905] -> w880
                  shift-left: w886 -> [w904]
                  n304 = Concatenate Strings(w904, w907, " (V)", "\t") -> (w905:string)
                }
                n305 = for {
                  shift-right: [w911] -> w888
                  shift-left: w891 -> [w912]
                  tunnel: w892 -> [w909] mode=indexing
                  n306 = Concatenate Strings(w912, w909, "\t") -> (w911:string)
                }
                n307 = for {
                  tunnel: w885 -> [w902] mode=indexing
                  shift-right: [w900] -> w884
                  shift-left: w880 -> [w899]
                  n308 = Concatenate Strings(w899, w902, " (I)", "\t") -> (w900:string)
                }
                n309 = Get Date/Time String() -> (date string=w897:string)  [unwired: 3 in, 1 out]
                n310 = Format Date/Time String() -> (date/time string=w879:string)  [unwired: 3 in]
                n311 = Build Path(base path=path "D:/Log_data/SC_LOG_HEADERS", name or relative path=w897) -> (appended path=w896:path)
                n312 = Concatenate Strings("Time\t", w889, w888, "Temp A\tTemp B\tHeater Power\tSetpoint\t", w884, "Time in seconds\tTime per cycle\t", w879, "\r\n") -> (w881:string)
                n313 = call <vilib>:"Write Spreadsheet String.vi"("append to file? (new file:F)"=TRUE, "spreadsheet string"=w881, "file path (dialog if empty)"=w896) -> ()  [unwired: 7 in, 2 out]
              }
            }
            n314 = Build Path(base path=path "D:/Log_data/SC_LOG", name or relative path=w869) -> (appended path=w868:path)
            n315 = Format Date/Time String() -> (date/time string=w873:string)  [unwired: 3 in]
            n316 = Array To Spreadsheet String(array=w875, 3:"%.3f" ("format string")) -> (spreadsheet string=w871:string)  [unwired: 1 in]
            n317 = Concatenate Strings(w873, "\t", w871) -> (w867:string)
            n318 = call <vilib>:"Write Spreadsheet String.vi"("append to file? (new file:F)"=TRUE, "spreadsheet string"=w867, "file path (dialog if empty)"=w868) -> ()  [unwired: 7 in, 2 out]
          }
          frame #7 {
            # "Status is True if ANY (armed)\ncondition is met"
            # "Detector P. Alert"
            # "Uninteruptable\n Power Supply Alert"
            # "Temp. Warning"
            # "Arms"
            # "Comm. Alert"
            # "Temperature Alert"
            # "Alarm conditions (Temp)"
            # "Check Alarms and Warnings"
            n319 = Unbundle By Name(w966) -> ("error out.status"=w948:bool)
            "NI mod 2&3 status" <- w948
            n320 = Unbundle By Name(w979) -> ("error out.status"=w977:bool)
            "LakeShore status" <- w977
            n321 = Unbundle By Name(w981) -> ("error out.status"=w976:bool)
            "CAEN 1 status" <- w976
            n322 = Unbundle By Name(w980) -> ("error out.status"=w975:bool)
            "CAEN 2 status" <- w975
            n323 = Unbundle By Name(w978) -> ("error out.status"=w974:bool)
            "NI mod1 (P) status" <- w974
            n324 = Build Array(w977, w976, w975, w974, w948) -> (w949:bool[])
            n325 = Build Array("LakeShore", "CAEN 1", "CAEN 2", "NI mod 2&3", "NI mod 1") -> (w944:bool[])
            n326 = call "check_ups.vi"() -> ("Error: no voltages read"=w928:bool, "Timestamp last measured"=→"Timestamp last \nmeasured (UPS)":timestamp, "Minimum input voltage measured"=w938:dbl)  [unwired: 8 in, 1 out]
            "Minimum input voltage measured" <- w938
            n327 = property on="Det.P input #" class="DigNum (strict)"() -> ("Value"=w964:i32)  [unwired: 2 in, 2 out]
            n328 = Or Array Elements(Boolean array=w949) -> (logical OR=→"Comm. status":bool)
            n329 = for {
              tunnel: w949 -> [w984] mode=indexing
              tunnel: w944 -> [w983] mode=indexing
              tunnel: [w982] -> w943 mode=indexing
              n330 = And(x=w984, y=w983) -> (x .and. y?=w982:bool)
            }
            n331 = Index Array(array=w965, index=w964) -> (element=w961:dbl)
            n332 = Less?(x=w938, y="UPS Voltage \nLower Threshold") -> (x < y?=w930:bool)
            n333 = Equal?(x=w938, y=-1.0) -> (x = y?=w929:bool)
            n334 = Less?(x=w961, y="Underpressure threshold") -> (x < y?=w959:bool)
            n335 = Build Array(w930, w929, w928) -> (w927:bool[])
            n336 = Or Array Elements(Boolean array=w943) -> (logical OR=w933:bool)
            n337 = Greater?(x=w961, y="Overpressure threshold") -> (0:w960:bool)
            n338 = Or(x=w960, y=w959) -> (x .or. y?=w958:bool)
            "Det. P. warning" <- w958
            n339 = Or Array Elements(Boolean array=w927) -> (logical OR=w926:bool)
            "Warning" <- w926
            n340 = And(x="UPS", y=w926) -> (x .and. y?=w932:bool)
            n341 = And(x=w958, y="Detector Pressure") -> (x .and. y?=w934:bool)
            n342 = Build Array("T 1", "T 2", "T 3", "T 4", "T 5", "T 6") -> (w924:bool[])
            n343 = for {
              tunnel: w923 -> [w985] mode=indexing
              tunnel: w924 -> [w988] mode=indexing
              tunnel: [w987] -> w935 mode=indexing
              tunnel: [w986] -> w950 mode=indexing
              n344 = Less?(x=w985, y="Low Temp threshold") -> (x < y?=w990:bool)
              n345 = Greater?(x=w985, y="High Temp threshold") -> (0:w989:bool)
              n346 = Or(x=w990, y=w989) -> (x .or. y?=w986:bool)
              n347 = And(x=w988, y=w986) -> (x .and. y?=w987:bool)
            }
            n348 = Index Array(array=w950) -> (element #1=→"Boolean":bool, element #2=→"Boolean 2":bool, element #3=→"Boolean 3":bool, element #4=→"Boolean 4":bool, element #5=→"Boolean 5":bool, element #6=→"Boolean 6":bool)  [unwired: 6 in]
            n349 = Build Array (concatenate)(w935, w934, w933, w932) -> (w931:bool[])
            n350 = Or Array Elements(Boolean array=w931) -> (logical OR=w925:bool)
            "Alarm state" <- w925
          }
          frame #8 {
            # "Testing alarm will not interfere"
            # "Act on alarm"
            n351 = Or(x="Test alarm", y=w999) -> (x .or. y?=w1000:bool)
            n352 = case shown="True" w1000 {
              tunnel: "Test alarm" -> [_ w1007]
              tunnel: w997 -> [_ w1015]
              tunnel: w993 -> [_ w1014]
              tunnel: w996 -> [w1003 w1005]
              tunnel: "Alarm\nMaster switch" -> [_ w1012]
              tunnel: [w1003 w1006] -> w994
              frame False {
                # "Timer stays at previous value"
              }
              frame True {
                n353 = Get Date/Time In Seconds() -> (seconds since 1Jan1904=w1019:timestamp)
                n354 = case shown="True" "\"Sound\" alarm" {
                  frame False {
                  }
                  frame True {
                    n355 = call <vilib>:"Beep.vi"("duration (msec)"=u32 1000, "frequency (Hz)"="Sound alarm\nFrequency (Hz)") -> ()  [unwired: 10 in]
                  }
                }
                n356 = To Double Precision Float(number=w1019) -> (double precision float=w1016:dbl)
                n357 = Multiply(x="Repeat Alarm SMS\nevery N minutes", y=60.0) -> (x*y=w1008:dbl)
                n358 = Subtract(x=w1016, y=w1005) -> (x-y=w1011:dbl)
                n359 = Greater?(x=w1011, y=w1008) -> (0:w1013:bool)
                n360 = And(x=w1012, y=w1013) -> (x .and. y?=w1010:bool)
                n361 = Or(x=w1007, y=w1010) -> (x .or. y?=w1009:bool)
                n362 = case shown="True" w1009 {
                  tunnel: w1007 -> [_ w1034]
                  tunnel: w1015 -> [_ w1042]
                  tunnel: w1014 -> [_ w1023]
                  tunnel: [w1022 w1032] -> w1006
                  tunnel: w1005 -> [w1022 w1031]
                  frame False {
                    # "Alarm not armed, or defined time has not yet passed"
                  }
                  frame True {
                    # "Average T in Det."
                    n363 = local read "Det.P input #"() -> (w1047:i32)
                    n364 = case shown="True" w1034 {
                      tunnel: ["Error encountered inXAMS! Status:" "TESTING the XAMS alarm. Status:"] -> w1041
                      tunnel: [w1051 w1054] -> w1032
                      tunnel: w1031 -> [_ w1054]
                      frame False {
                        n365 = Get Date/Time In Seconds() -> (seconds since 1Jan1904=w1052:timestamp)
                        n366 = To Double Precision Float(number=w1052) -> (double precision float=w1051:dbl)
                      }
                      frame True {
                      }
                    }
                    n367 = for {
                      tunnel: w1023 -> [w1056] mode=indexing
                      tunnel: [w1063] -> w1026 mode=indexing
                      i -> [w1057]
                      n368 = Format Into String(format string="%.0f", w1057) -> (resulting string=w1061:string)  [unwired: 2 in, 1 out]
                      n369 = Format Into String(format string="%.1f", w1056) -> (resulting string=w1059:string)  [unwired: 2 in, 1 out]
                      n370 = Concatenate Strings("\n" ("format string"), w1061, "     " ("format string"), w1059) -> (w1063:string)
                    }
                    n371 = Index Array(array=w1042, index=w1047) -> (element=w1043:dbl)
                    n372 = Array Size(array=w1023) -> (size(s)=w1045:i32)
                    n373 = Add Array Elements(numeric array=w1023) -> (sum=w1046:dbl)
                    n374 = Format Into String(format string="%.3f", w1043) -> (resulting string=w1037:string)  [unwired: 2 in, 1 out]
                    n375 = Divide(x=w1046, y=w1045) -> (x/y=w1035:dbl)
                    n376 = Format Date/Time String() -> (date/time string=w1039:string)  [unwired: 3 in]
                    n377 = Format Into String(format string="%.2f", w1035) -> (resulting string=w1024:string)  [unwired: 2 in, 1 out]
                    n378 = Concatenate Strings(w1041, "\nDate/time: ", w1039, "\nDetector Pressure: ", w1037, " bar", "\nDetector Temperatures (°C):", "\nCh:   Temp:" ("format string"), w1026, "\nAverage detector temperature: ", w1024) -> (w1030:string)
                    "Alarm (or test) message" <- w1030
                    n379 = for {
                      tunnel: w1030 -> [w1050]
                      tunnel: "Phone numbers" -> [w1049] mode=indexing
                      n380 = call "send_sms.vi"("Message content"=w1050, "Phone number"=w1049) -> ("standard error"=→"SMS error":string)  [unwired: 8 in, 1 out]
                    }
                  }
                }
              }
            }
            n381 = And(x="Shut off heater \nif Alarm is active", y=w999) -> (x .and. y?=w1001:bool)
            "Alarm active 2" <- "Alarm\nMaster switch"
          }
          frame #9 {
            # "Daily e-mail"
            n382 = Get Date/Time In Seconds() -> (seconds since 1Jan1904=w1078:timestamp)
            n383 = To Double Precision Float(number=w1078) -> (double precision float=w1077:dbl)
            n384 = Get Date/Time String(want seconds? (F)=FALSE) -> (time string=w1080:string)  [unwired: 2 in, 1 out]
            n385 = Subtract(x=w1077, y=w1070) -> (x-y=w1076:dbl)
            n386 = Equal?(x=w1080, y="Send status email at time:") -> (x = y?=w1073:bool)
            n387 = Greater?(x=w1076, y=62) -> (0:w1072:bool)
            n388 = Build Array("Send daily email?", w1073, w1072) -> (w1071:bool[])
            n389 = And Array Elements(Boolean array=w1071) -> (logical AND=w1067:bool)
            n390 = Or(x="Send status email now", y=w1067) -> (x .or. y?=w1068:bool)
            n391 = case shown="True" w1068 {
              tunnel: w1065 -> [_ w1085]
              tunnel: w1083 -> [_ w1102]
              tunnel: w1082 -> [_ w1111]
              tunnel: w1070 -> [w1084 _]
              tunnel: [w1084 w1097] -> w1069
              frame False {
              }
              frame True {
                # "Average T in Det."
                n392 = Not Equal To 0?(x="Number of Bonus lines") -> (x != 0?=w1090:bool)
                n393 = case shown="True" w1090 {
                  tunnel: [w1122 w1125] -> w1091
                  tunnel: "Number of Bonus lines" -> [_ w1128]
                  frame False {
                    n394 = Build Array("\n[Flavor text module inactive]") -> (w1122:string[])
                  }
                  frame True {
                    n395 = Build Path(base path=path "C:/Users/xams/Desktop/New XAMS Slow Control", name or relative path="cool_beans.txt") -> (appended path=w1129:path)
                    n396 = call-poly <vilib>:"Read Delimited Spreadsheet.vi"("file path (dialog if empty)"=w1129) -> ("all rows"=w1132:string[][])  [unwired: 9 in, 5 out]
                    n397 = Array Size(array=w1132) -> (size(s)=w1134:i32[])
                    n398 = Index Array(array=w1134) -> (element=w1133:i32)  [unwired: 1 in]
                    n399 = for {
                      N: w1128 -> [_]
                      tunnel: w1133 -> [w1139]
                      tunnel: w1132 -> [w1138]
                      tunnel: [w1135] -> w1126 mode=indexing
                      n400 = Random Number (0-1)() -> (number: 0 to 1=w1142:dbl)
                      n401 = Multiply(x=w1139, y=w1142) -> (x*y=w1141:dbl)
                      n402 = Round To Nearest(number=w1141) -> (nearest integer value=w1140:dbl)
                      n403 = Index Array(array=w1138, index (row)=w1140) -> (element=w1136:string[])  [unwired: 1 in]
                      n404 = Concatenate Strings("\n", w1136) -> (w1135:string)
                    }
                    n405 = Concatenate Strings("\n\nCool beans of the day: ", w1126) -> (w1124:string)
                    n406 = Build Array(w1124) -> (w1125:string[])
                  }
                }
                n407 = local read "Det.P input #"() -> (w1112:i32)
                n408 = for {
                  tunnel: [w1151] -> w1104 mode=indexing
                  tunnel: w1085 -> [w1143] mode=indexing
                  i -> [w1144]
                  n409 = Format Into String(format string="%.0f", w1144) -> (resulting string=w1148:string)  [unwired: 2 in, 1 out]
                  n410 = Format Into String(format string="%.2f", w1143) -> (resulting string=w1146:string)  [unwired: 2 in, 1 out]
                  n411 = Concatenate Strings("\nCh: " ("format string"), w1148, ", Temp: " ("format string"), w1146, "°C." ("format string")) -> (w1151:string)
                }
                n412 = Array Size(array=w1085) -> (size(s)=w1120:i32)
                n413 = Add Array Elements(numeric array=w1085) -> (sum=w1121:dbl)
                n414 = Index Array(array=w1111, index=w1112) -> (element=w1109:dbl)
                n415 = Divide(x=w1121, y=w1120) -> (x/y=w1118:dbl)
                n416 = Format Into String(format string="%.3f", w1109) -> (resulting string=w1107:string)  [unwired: 2 in, 1 out]
                n417 = Format Into String(format string="%.2f", w1118) -> (resulting string=w1101:string)  [unwired: 2 in, 1 out]
                n418 = Select(t="ACTIVE!!!!!", s=w1102, f="inactive.") -> (s? t:f=w1114:string)
                n419 = Concatenate Strings("Hello, XAMS teammembers.", "\n\nThe alarm is currently ", w1114, "\n\nThe latest detector pressure is: ", w1107, " bar." ("format string"), "\nTemperatures inside the detector are:", w1104, "\nThe average detector temperature is ", w1101, "°C." ("format string"), "\n\nThank you for doing your best today, once again!\nRegards, SC.", w1091) -> (w1096:string)
                "Status email preview" <- w1096
                n420 = call "custom_email_program.vi"("mail server"="smtp.nikhef.nl", "return address"="return address", "message"=w1096, "subject ([No Subject])"="XAMS daily status email.", "Email Adresses"="Email Addresses") -> ("error out"=w1088:errorcluster)  [unwired: 6 in]
                n421 = Unbundle By Name(w1088) -> ("code"=→"Email error":i32, "source"=→"source":string)
                n422 = Get Date/Time In Seconds() -> (seconds since 1Jan1904=w1098:timestamp)
                n423 = To Double Precision Float(number=w1098) -> (double precision float=w1097:dbl)
              }
            }
          }
        }
        n424 = Decrement(x="Cycles to execute") -> (x-1=w287:dbl)
        n425 = Decrement(x=w287) -> (x-1=w286:dbl)
        n426 = Greater?(x=w270, y=w286) -> ()  [unwired: 1 out]
        n427 = Decrement(x="Clear data every N cycles") -> (x-1=w267:dbl)
        n428 = Greater?(x=w270, y=w267) -> (0:w269:bool)
        n429 = And(x="Auto-clear data?", y=w269) -> (x .and. y?=w272:bool)
        n430 = Or(x=w272, y="Clear data") -> (x .or. y?=w274:bool)
        n431 = case shown="False" w274 {
          tunnel: w285 -> [w315 _]
          tunnel: [w315 dbl[][] []] -> w284
          tunnel: w283 -> [w314 _]
          tunnel: [w314 w321] -> w282
          tunnel: w281 -> [w313 _]
          tunnel: [w313 w321] -> w280
          tunnel: w279 -> [w312 _]
          tunnel: [w312 w319] -> w278
          tunnel: w277 -> [w311 _]
          tunnel: [w311 w317] -> w276
          tunnel: w270 -> [w310 _]
          tunnel: [w310 0] -> w271
          frame False {
          }
          frame True {
            w321 = 0.0
            n432 = Get Date/Time In Seconds() -> (seconds since 1Jan1904=w318:timestamp)
            n433 = To Double Precision Float(number=w318) -> (double precision float=w320:dbl)
            n434 = Build Array(w318) -> (w317:timestamp[])
            n435 = Build Array(w320, w320) -> (w319:dbl[])
          }
        }
        n436 = Or(x=FALSE, y="stop") -> (x .or. y?=w307:bool)
        "Auto-clear" <- "Auto-clear data?"
      }
    }
    frame True {
    }
  }
  n437 = flat-sequence {
    tunnel: w20 -> [w1195]
    tunnel: w16 -> [w1186]
    tunnel: w15 -> [w1183]
    tunnel: w14 -> [w1178]
    tunnel: w7 -> [w1167]
    tunnel: w2 -> [w1164]
    frame #0 {
      w1191 = u16 2 items=["1"=1, "2"=2] ("Heater Output (1:1)")
      w1192 = u16 0 items=["Off", "Low (On)", "Medium", "High"] ("Range (0:Off)")
      # "Important icons! Always press STOP button when done \ninstead of force closing, otherwise these don't get executed"
      # "Turn off heater, shutdown COM"
      # "Error Handling and Post-Processing (EHaPP)"
      n438 = Unbundle(w1195) -> ("VISA resource name out"=w1194:refnum<visa-resource-name>, "error out"=w1193:errorcluster)
      n439 = Unbundle(w1186) -> ("VISA resource name out"=w1185:refnum<visa-resource-name>, "error out"=w1184:errorcluster)
      n440 = Unbundle(w1183) -> ("VISA resource name out"=w1182:refnum<visa-resource-name>, "error out"=w1181:errorcluster)
      n441 = Unbundle(w1178) -> ("task out"=w1176:refnum<k21>, "error out"=w1174:errorcluster)
      n442 = Unbundle(w1167) -> ("task out"=w1171:refnum<k21>, "error out"=w1169:errorcluster)
      n443 = Unbundle(w1164) -> ("task out"=w1163:refnum<k21>, "error out"=w1162:errorcluster)
      n444 = call <vilib>:"DAQmx Stop Task.vi"("task/channels in"=w1176, "error in"=w1174) -> ("task out"=w1175:refnum<k21>, "error out"=w1173:errorcluster)  [unwired: 12 in]
      n445 = call <vilib>:"DAQmx Stop Task.vi"("task/channels in"=w1171, "error in"=w1169) -> ("task out"=w1170:refnum<k21>, "error out"=w1168:errorcluster)  [unwired: 12 in]
      n446 = call <vilib>:"DAQmx Stop Task.vi"("task/channels in"=w1163, "error in"=w1162) -> ("task out"=w1161:refnum<k21>, "error out"=w1165:errorcluster)  [unwired: 12 in]
      n447 = call <instrlib>:"Configure Output Range and Manual Value.vi"("VISA resource name"=w1194, "Heater Output (1:1)"=w1191, "Range (0:Off)"=w1192, "Manual Output (0.00 %)"=0.0, "error in (no error)"=w1193) -> ("VISA resource name out"=w1189:refnum<visa-resource-name>, "error out"=w1188:errorcluster)  [unwired: 9 in]
      n448 = call <instrlib>:"Close.vi"("error in (no error)"=w1184, "VISA resource name"=w1185) -> ("error out"=w1180:errorcluster)  [unwired: 9 in]
      n449 = call <instrlib>:"Close.vi"("error in (no error)"=w1181, "VISA resource name"=w1182) -> ("error out"=w1179:errorcluster)  [unwired: 9 in]
      n450 = call <instrlib>:"Close.vi"("error in (no error)"=w1188, "VISA resource name"=w1189) -> ("error out"=w1187:errorcluster)  [unwired: 9 in]
      n451 = call <vilib>:"DAQmx Clear Task.vi"("task in"=w1175, "error in"=w1173) -> ("error out"=w1177:errorcluster)  [unwired: 13 in]
      n452 = call <vilib>:"DAQmx Clear Task.vi"("task in"=w1170, "error in"=w1168) -> ("error out"=w1172:errorcluster)  [unwired: 13 in]
      n453 = call <vilib>:"DAQmx Clear Task.vi"("task in"=w1161, "error in"=w1165) -> ("error out"=w1166:errorcluster)  [unwired: 13 in]
      n454 = call <vilib>:"Simple Error Handler.vi"("error in (no error)"=w1187) -> ()  [unwired: 4 in, 5 out]
      n455 = call <vilib>:"Simple Error Handler.vi"("error in (no error)"=w1180) -> ()  [unwired: 4 in, 5 out]
      n456 = call <vilib>:"Simple Error Handler.vi"("error in (no error)"=w1179) -> ()  [unwired: 4 in, 5 out]
      n457 = call <vilib>:"Simple Error Handler.vi"("error in (no error)"=w1177) -> ()  [unwired: 4 in, 5 out]
      n458 = call <vilib>:"Simple Error Handler.vi"("error in (no error)"=w1172) -> ()  [unwired: 4 in, 5 out]
      n459 = call <vilib>:"Simple Error Handler.vi"("error in (no error)"=w1166) -> ()  [unwired: 4 in, 5 out]
    }
  }
  n460 = Array Size(array=w30) -> (size(s)=w33:i32)
  n461 = Decrement(x=w33) -> (x-1=w32:i32)
  n462 = Index Array(array=w30, index #1=w32, index #2=1 ("index")) -> (element #1=w31:timestamp, element #2=w12:timestamp)
  n463 = To Double Precision Float(number=w31) -> (double precision float=w29:dbl)
  n464 = To Double Precision Float(number=w12) -> (double precision float=w28:dbl)
  n465 = Subtract(x=w29, y=w28) -> ()  [unwired: 1 out]
  "Started up?" <- w24
